vi "ConvertGoop1ToGoop3.vi"() -> (0 "error out":errorcluster)   [LabVIEW 2020]
uses:
  <resource>/Framework/Providers/Open_GDS/ClassProviders/Common/ConvertGoop2ToGoop3_SubVIs/ConvertGoop2ToGoop3_ClassInfo.ctl
  <resource>/Framework/Providers/Open_GDS/ClassProviders/Common/LvClass_class/GDSLvCLass_ClassSettingsType.ctl
  <resource>/Framework/Providers/Open_GDS/ClassProviders/Common/LvClass_class/GDSLvClass_PlugIn.ctl
  <resource>/Framework/Providers/Open_GDS/ClassProviders/Common/LvClass_class/GDSLvClass_PlugInTypes.ctl
  <vilib>/Utility/miscctls.llb/LVPositionTypeDef.ctl
  <vilib>/Utility/error.llb/DialogType.ctl
  <resource>/Framework/Providers/Open_GDS/ClassProviders/Provider_BaseClassInterface/CreateClassData.ctl
  <resource>/Framework/Providers/Open_GDS/ClassProviders/Provider_EndevoGOOP300/Templates/EndevoTemplateNames.ctl
  <resource>/Framework/Providers/Open_GDS/ClassProviders/Provider_EndevoGOOP300/ClassWriterGOOP300_class/ClassWriterGOOP300.lvclass
  <vilib>/picture/picture.llb/imagedata.ctl
  <resource>/Framework/Providers/Open_GDS/ClassProviders/Provider_EndevoGOOP300/EndevoProviderName.ctl
  <vilib>/regexp/Match Regular Expression.xnode
  <resource>/Framework/Providers/Open_GDS/ClassProviders/Provider_BaseClassInterface/ClassWriter_class/ClassWriter.lvclass
panel:
  in  "Cancel":bool
  in  "Next":bool
  out "Tab":T1(tab)
  in  "Current GOOP1 top directory":path
  out "Additional VIs that has been found\nand will be relinked:":i32
  out "GOOP1 classes found":string
  in  "VisToRelink":path[](array[path])
  in  "Project":path caption="This project will be created and have all classes added to it:"
  in  "Progress":i32(listbox)
  in  "Done":bool
  out "State":string
  # "1."
  # "Select Top folder to start a recursive search for GOOP1 classes and application VIs."
  # "2."
  # "These classes\nhave been found.\n\nDo you want to convert them?"
  # "3."
  # "Have you backed up all your VIs in the selected folder?"
  # "Have you checked that all files in\nthe selected folder are writeable?"
  # "Relinking VIs outside top folder?\nIf you want to relink any VIs to the new classes that are outside the selected top folder, add them to the list below"
  # "4."
  # "Save VI dialog boxes!?!\nIt might pop up dialog boxes that asks you to save VIs that will be unloaded from memory, JUST press cancel for those."
  # "Revert dialog boxes!?!\nIt might pop up dialog boxes that prompts that changes has been done on disk, JUST press cancel for those."
  # "5."
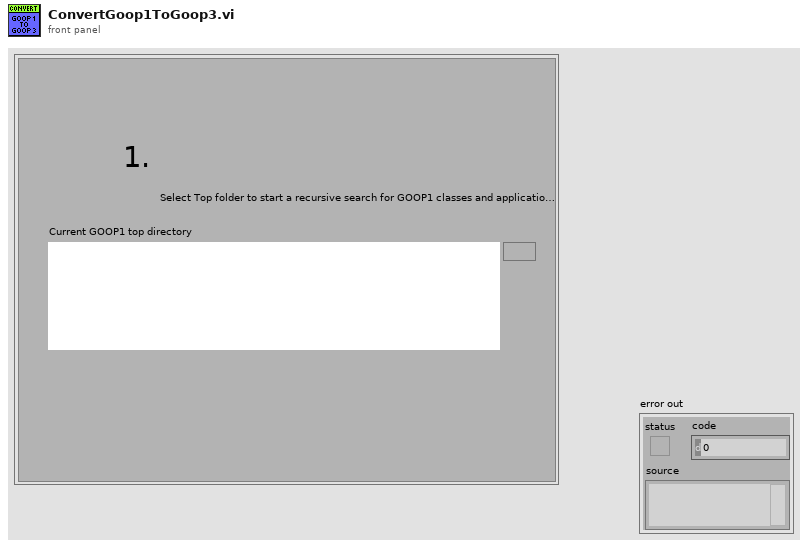
[diagram p1: front panel]
types:
  T1 = enum32{"GOOP2Dir", "ClassesFound", "BackedUp", "Start?", "Converting"}
  T2 = typedef "ConvertGoop2ToGoop3_ClassInfo.ctl" = cluster{"NoOfInheritance":i32, "LvClassPath":path, "ClassName":string, "ClassPrefix":string, "IsLLB":bool, "ClassFolder":path, "ViRefs":refnum<vi>[], "ClassRef":refnum<vi>, "InheritsFrom":path, "RootClass":path, "ViPathes":path[], "AllInheritanceClasses":string[], "TemplateVersionUsed":string, "UsingClassAttributes":bool, "ClassSettings":T3, "HeaderIcon":u8[][]}
  T3 = typedef "GDSLvCLass_ClassSettingsType.ctl" = cluster{"ClassProviderName":string, "ClassTemplateUsed":string, "ClassTemplateVersion":string, "ClassDescription":string, "PlugIns":T4[], "ConnectorPanePattern":string}
  T4 = typedef "GDSLvClass_PlugIn.ctl" = cluster{"Type":T5, "ID":string, "Version":string, "Path":path, "Name":string, "Data":variant}
  T5 = typedef "GDSLvClass_PlugInTypes.ctl" = enum16{"DesignPattern", "MethodTypes"}
  T6 = typedef "LVPositionTypeDef.ctl" = cluster{"Left":i32, "Top":i32}
  T7 = cluster{"TopFolderPath":path, "Classes":T2[], "SetToDynamicDispatch":refnum<vi>[], "error":errorcluster, "Project":path, "ProjectRef":refnum<vi>, "My Computer":refnum<vi>, "AppRef":refnum<vi>, "VIsToRelink":refnum<vi>[], "VIsToRelink(Paths)":path[], "CallParentMethod":cluster{"VIRef":refnum<vi>, "Position":T6}[], "CopyClasses":path, "TemplateVersions":string[], "LLBsToDelete":path[]}
  T8 = enum32{"GOOP2Dir", "ClassesFound", "GOOP3Dir", "Start?", "Converting"}
  T9 = typedef "EndevoTemplateNames.ctl" = enum16{"BaseTemplate", "SubTemplate", "BaseTemplate_4x4x4", "SubTemplate_4x4x4", "SingletonTemplate"}
  T10 = typedef "ClassWriter.lvclass/CreateClassData.ctl" = cluster{"ClassName":string, "ClassFolder":path, "ClassDescription":string, "ClassTemplateOptions":string, "BaseClass(ProjectStringPath or LvClassFilePath)":variant, "ExtraCreateParameters":variant, "FolderSuffix":string}
  T11 = enum32{"invalid scope", "public", "private", "protected"}
  T12 = typedef "imagedata.ctl" = cluster{"image type":i32, "image depth":i32, "image":u8[], "mask":u8[], "colors":u32[], "Rectangle":cluster{"left":i16, "top":i16, "right":i16, "bottom":i16}}
  T13 = typedef "EndevoProviderName.ctl" = enum16{"EndevoGOOP300"}
  T14 = typedef "DialogType.ctl" = u16
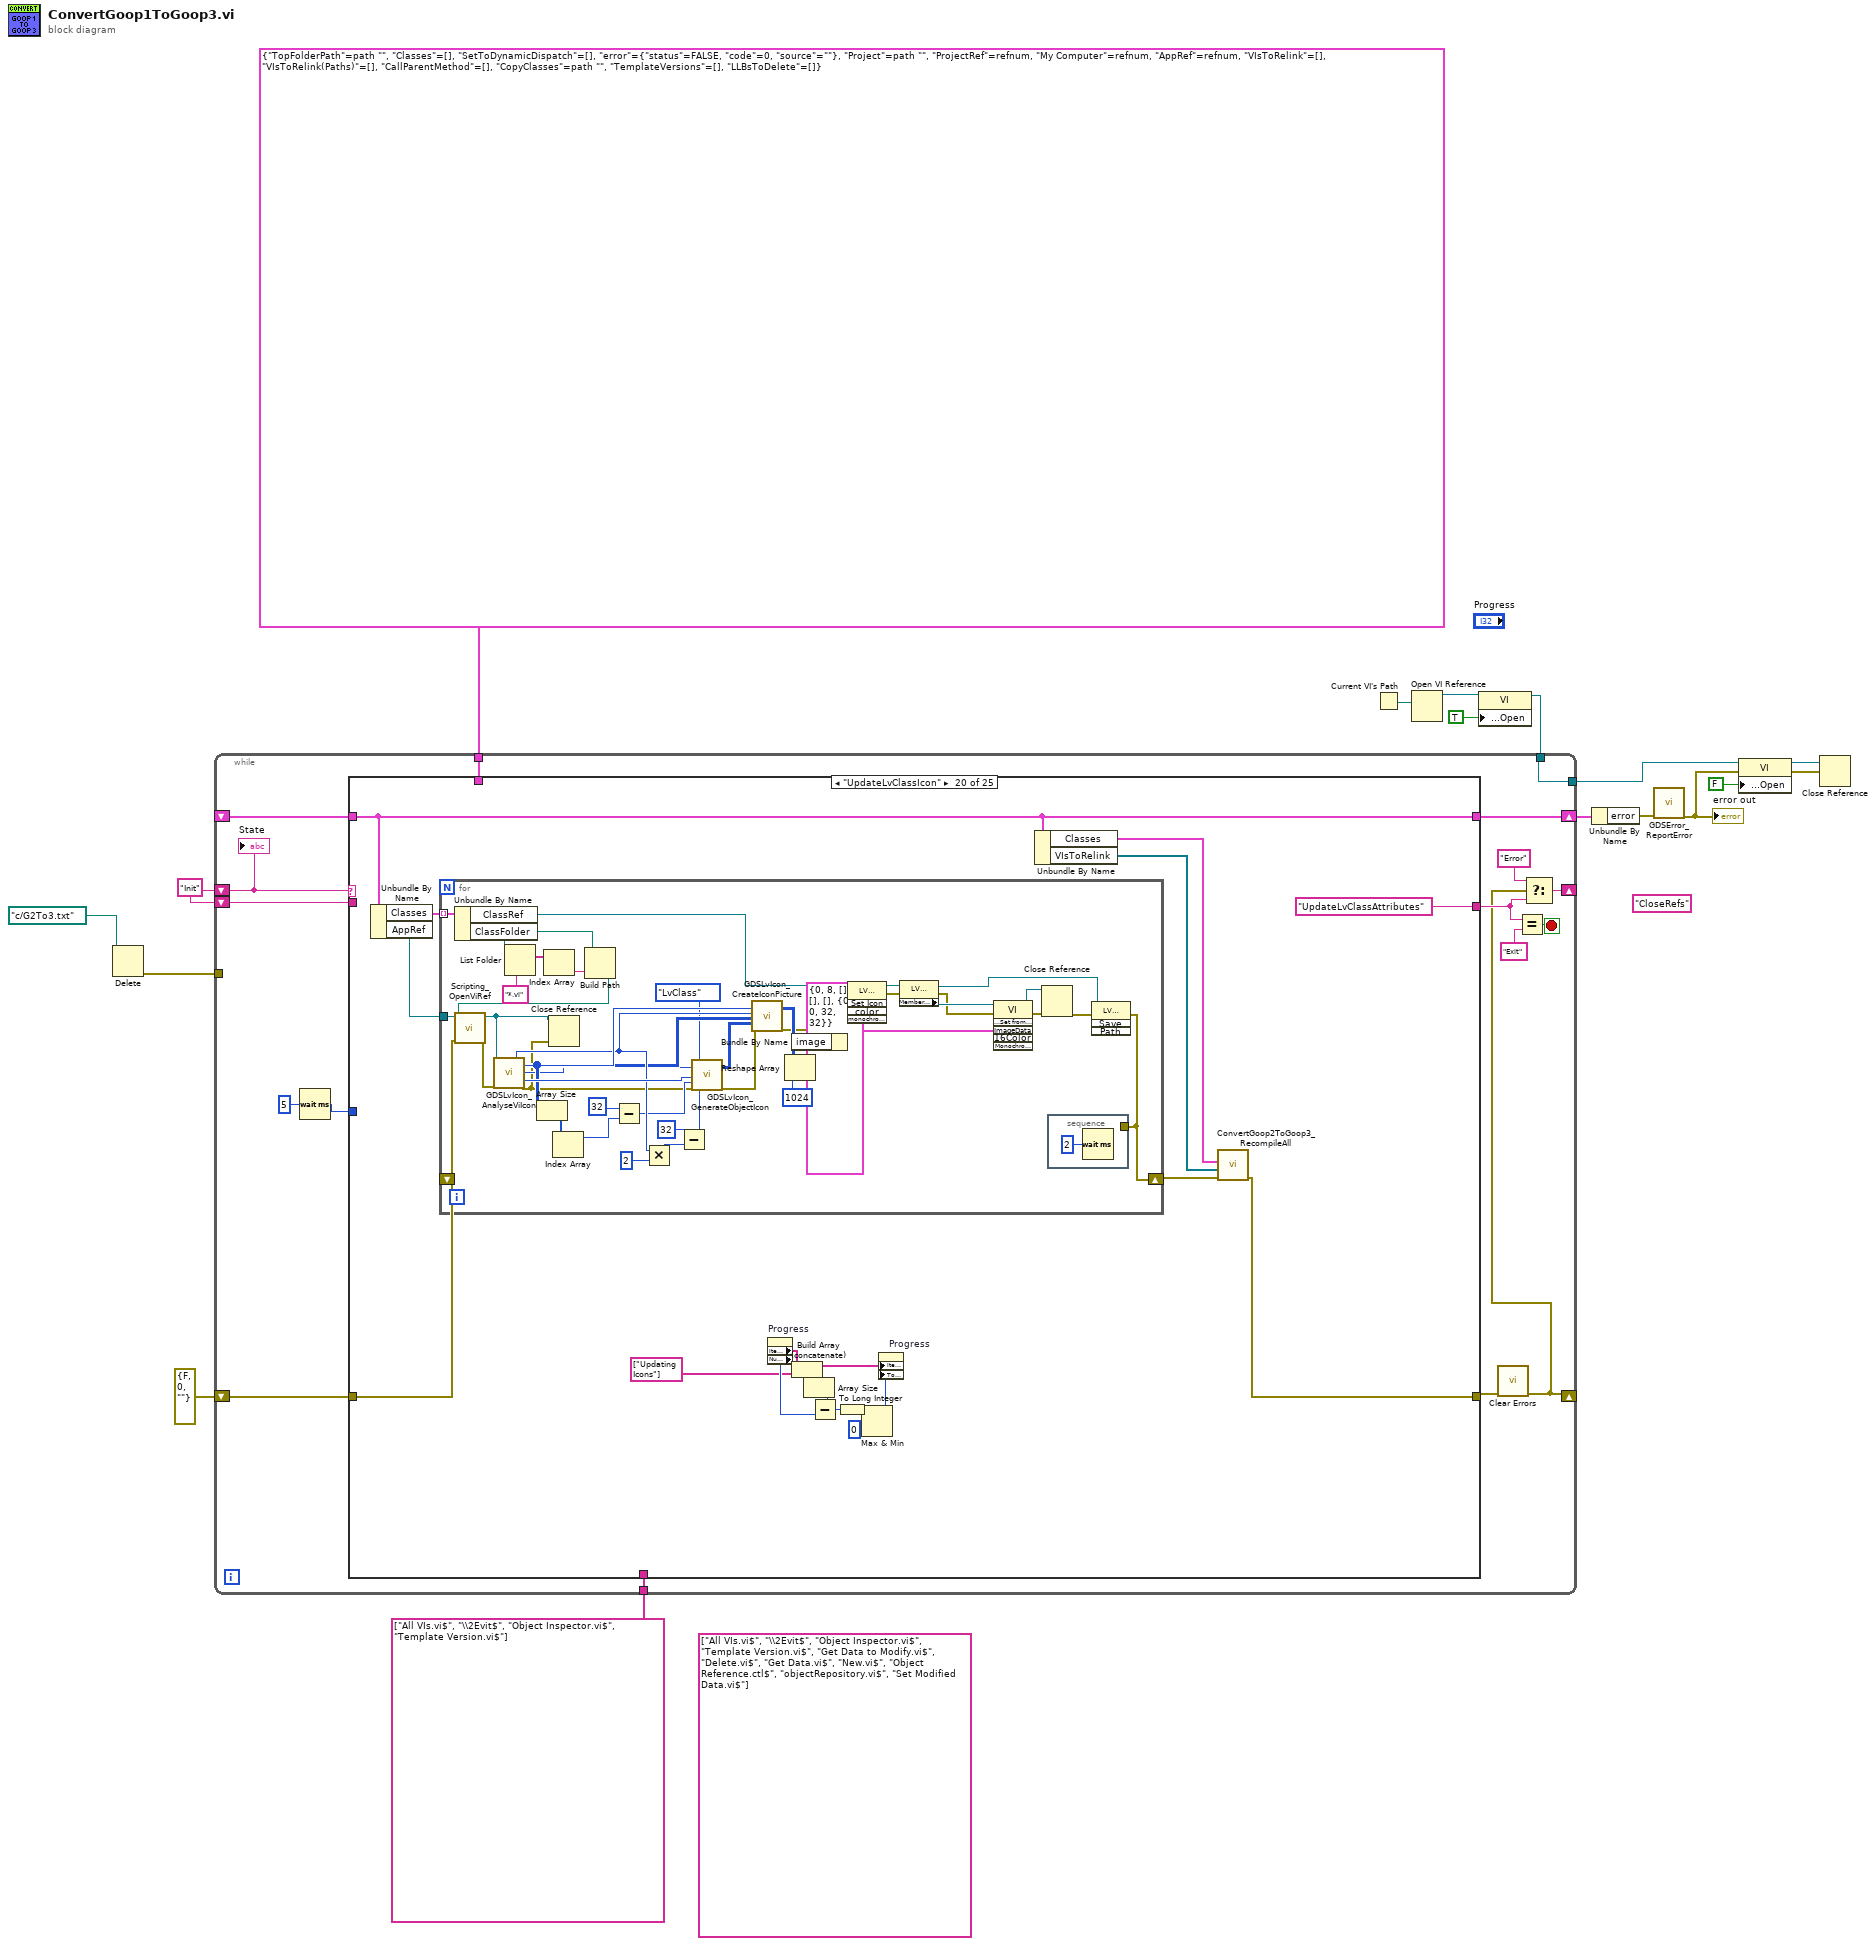
[diagram p0: block diagram]
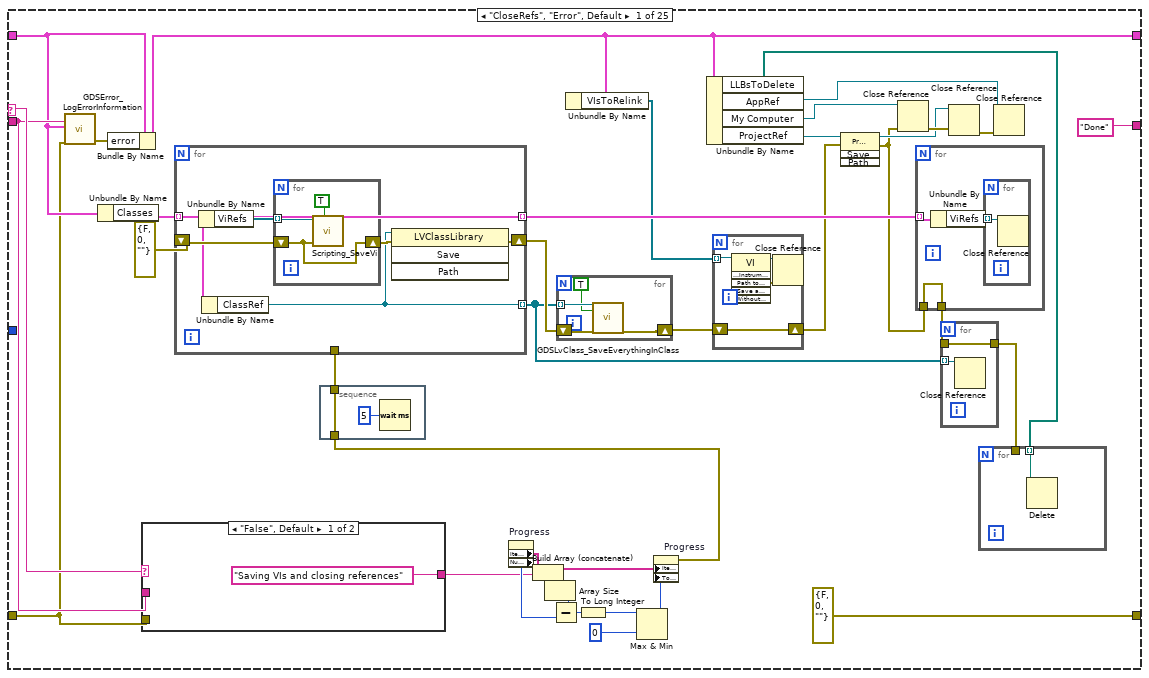
[diagram p2: hidden frame]
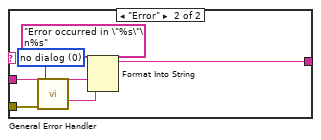
[diagram p3: hidden frame]
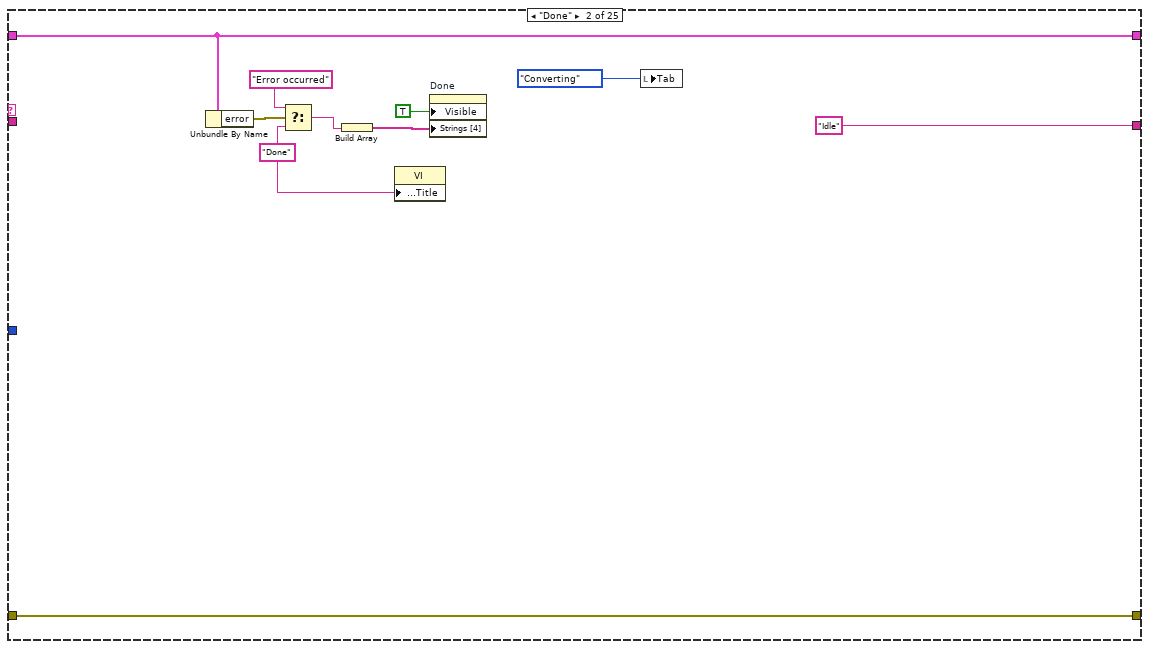
[diagram p4: hidden frame]
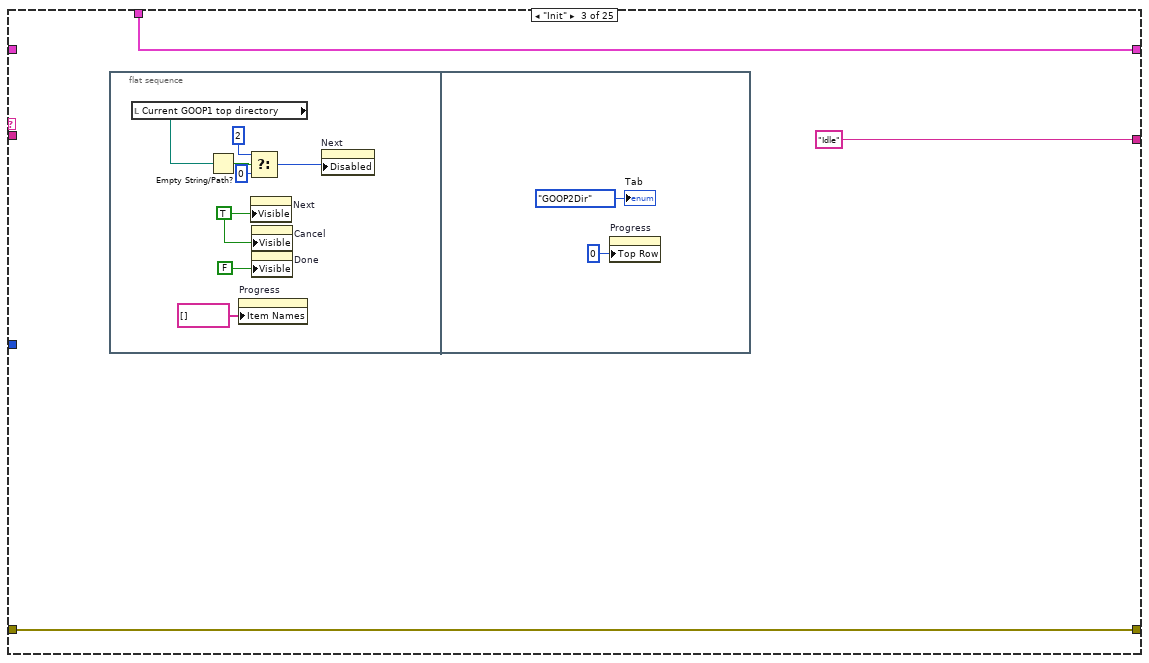
[diagram p5: hidden frame]
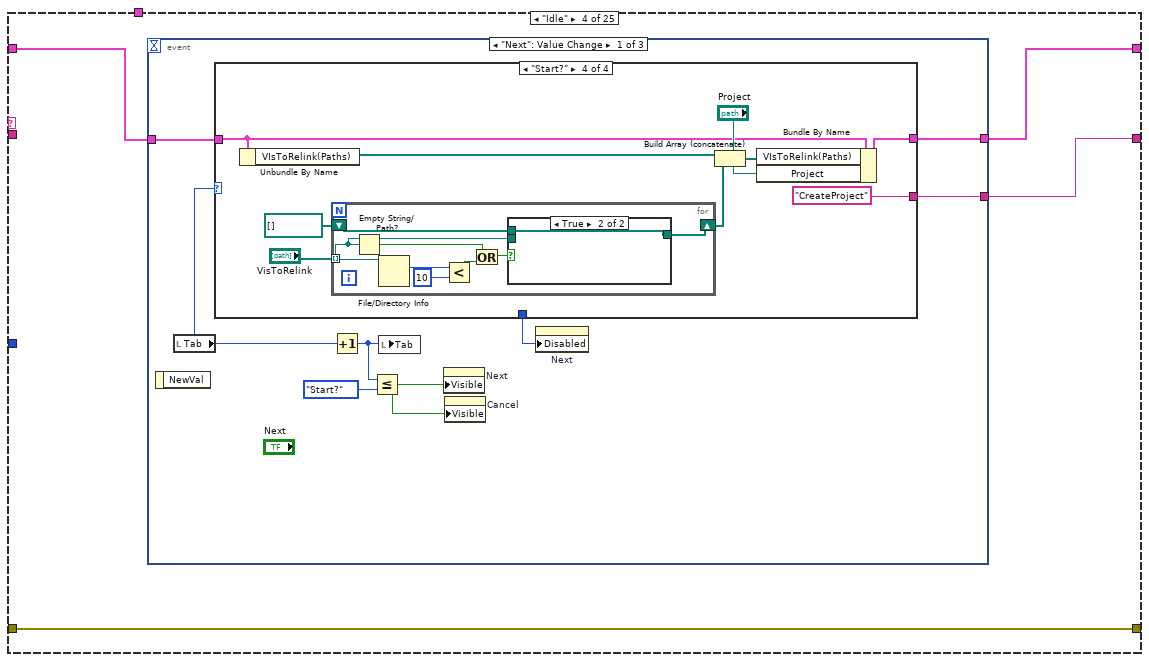
[diagram p6: hidden frame]
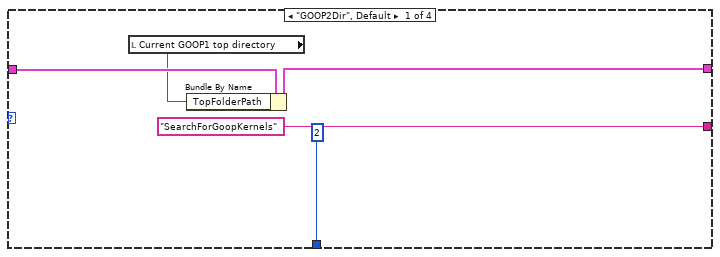
[diagram p7: hidden frame]
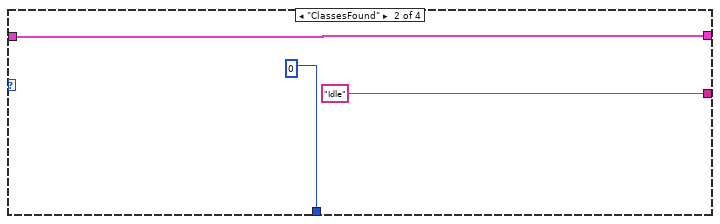
[diagram p8: hidden frame]
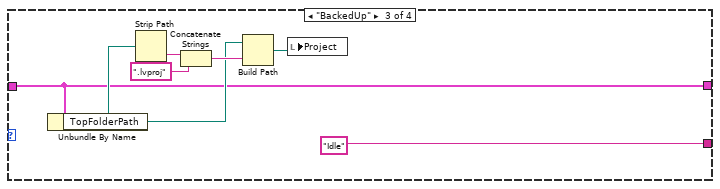
[diagram p9: hidden frame]
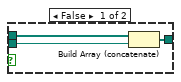
[diagram p10: hidden frame]
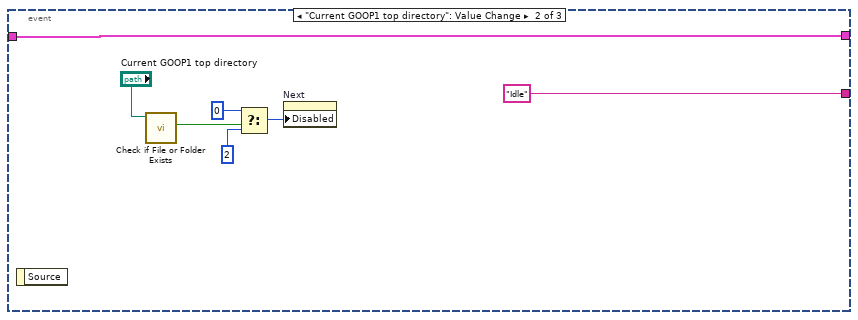
[diagram p11: hidden frame]
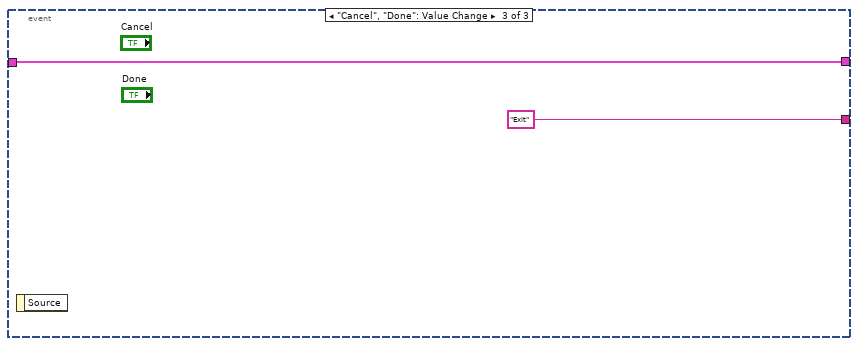
[diagram p12: hidden frame]
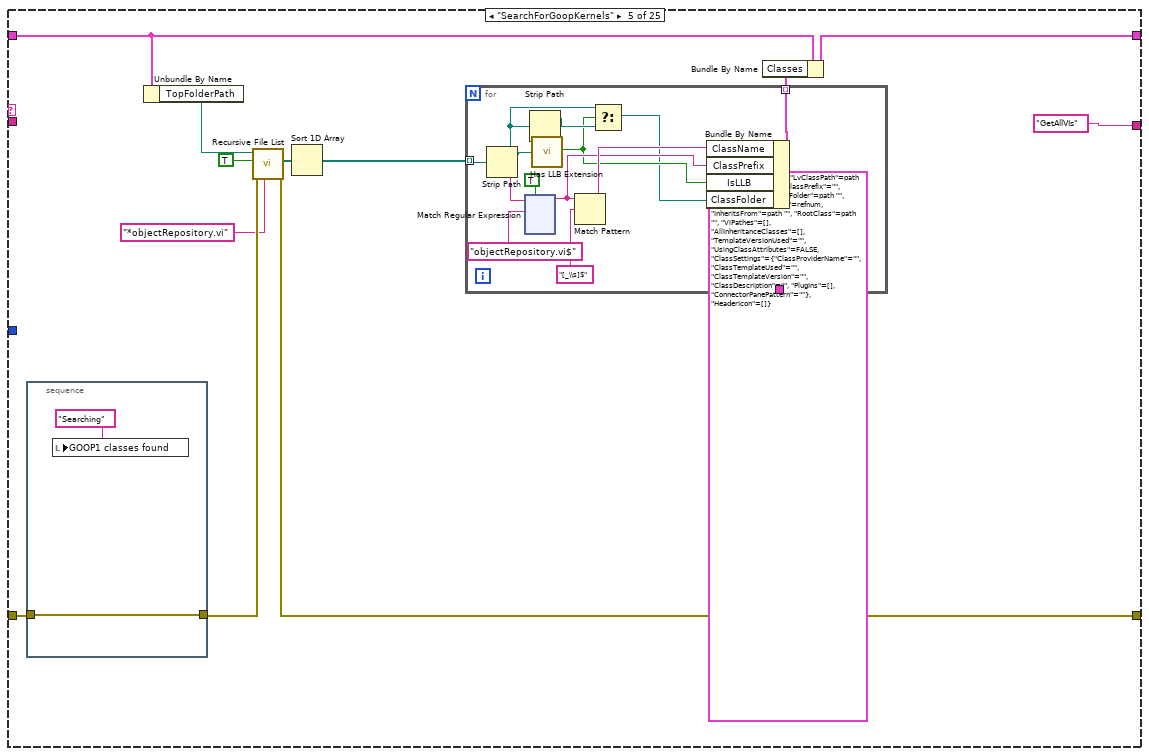
[diagram p13: hidden frame]
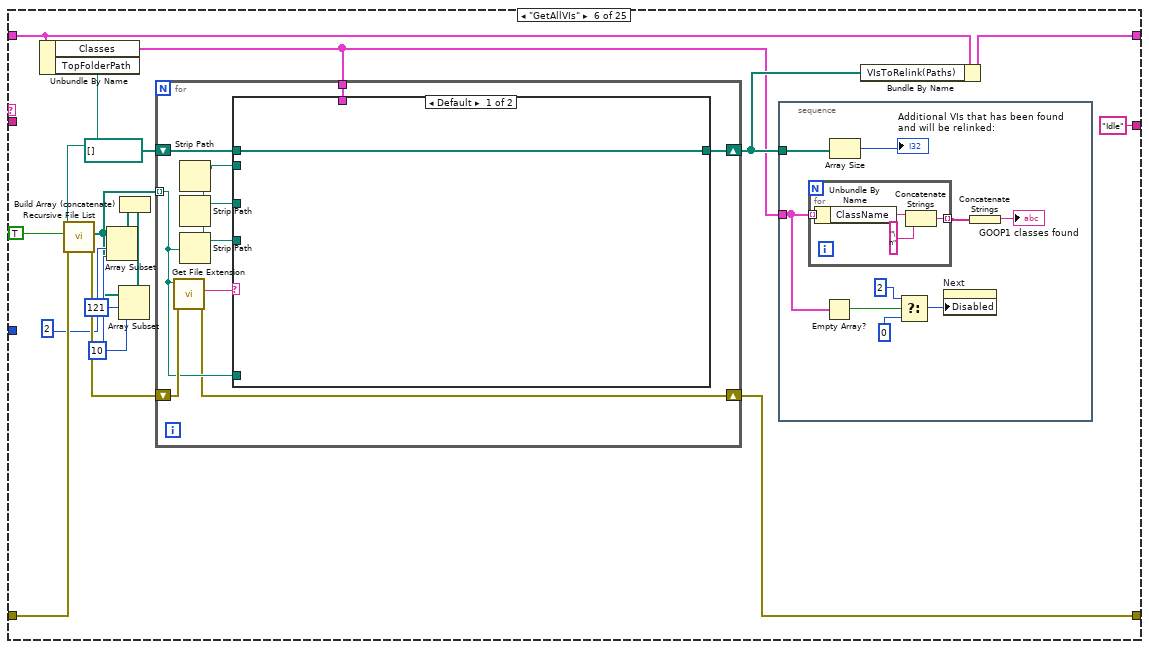
[diagram p14: hidden frame]
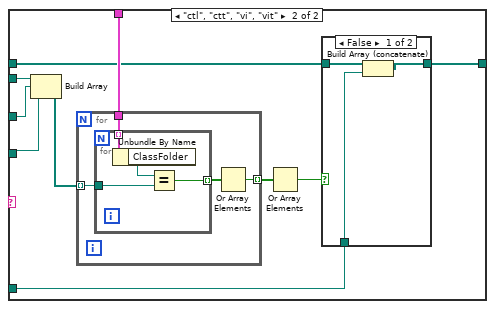
[diagram p15: hidden frame]
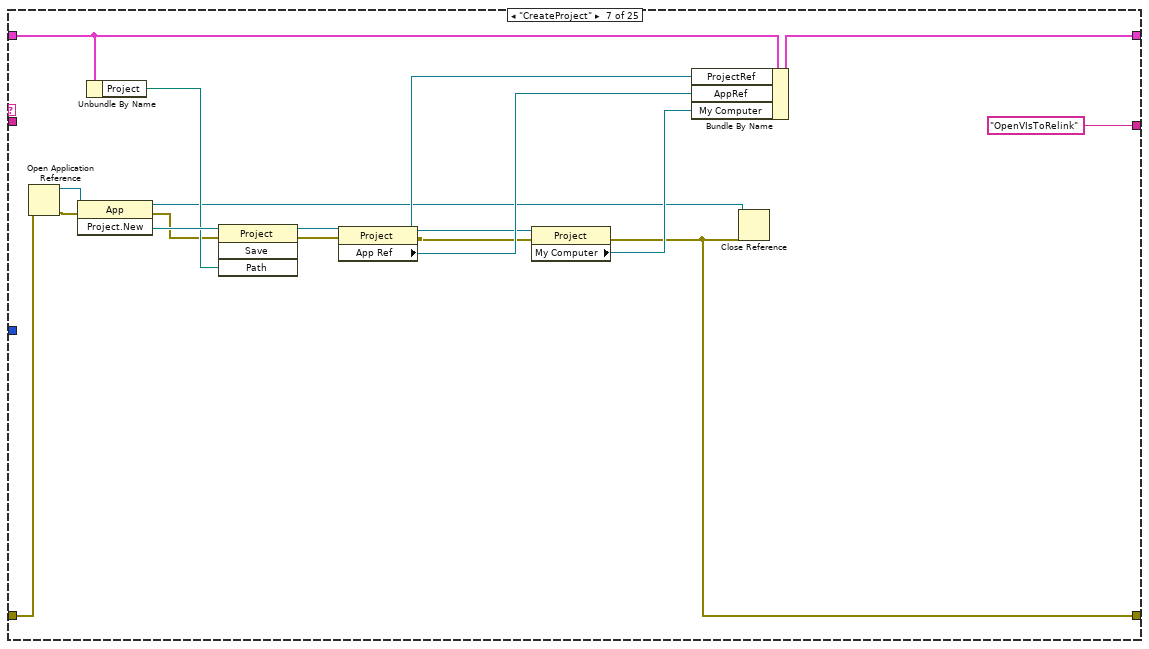
[diagram p17: hidden frame]
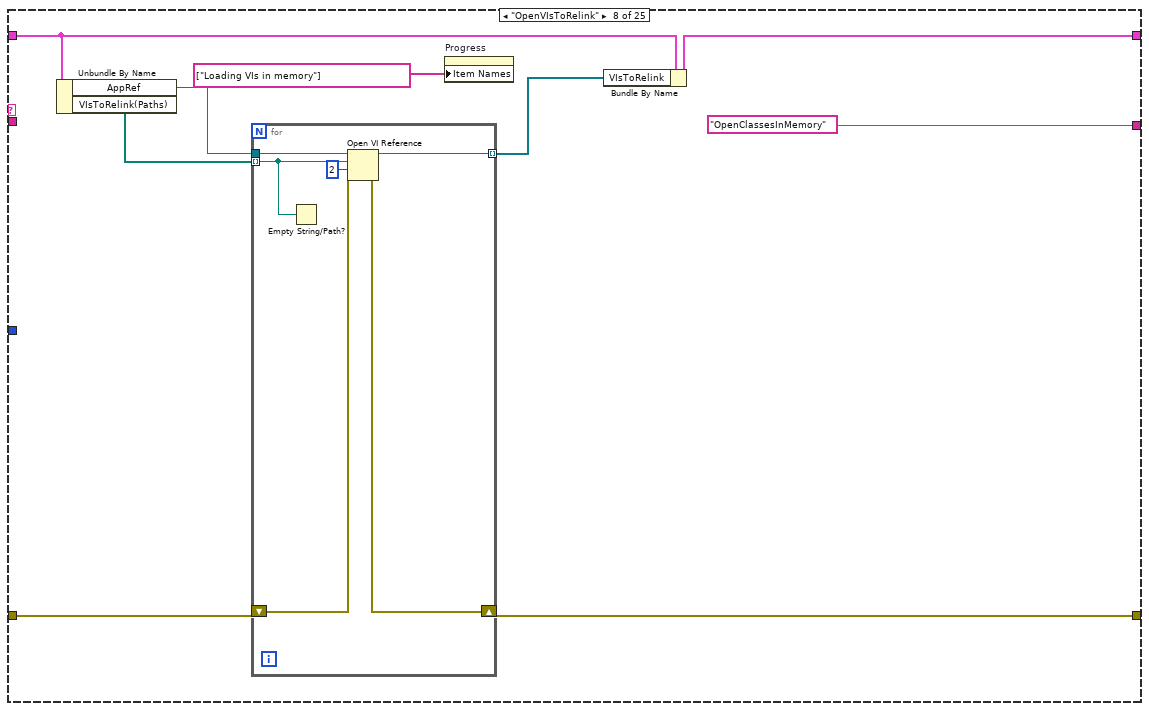
[diagram p18: hidden frame]
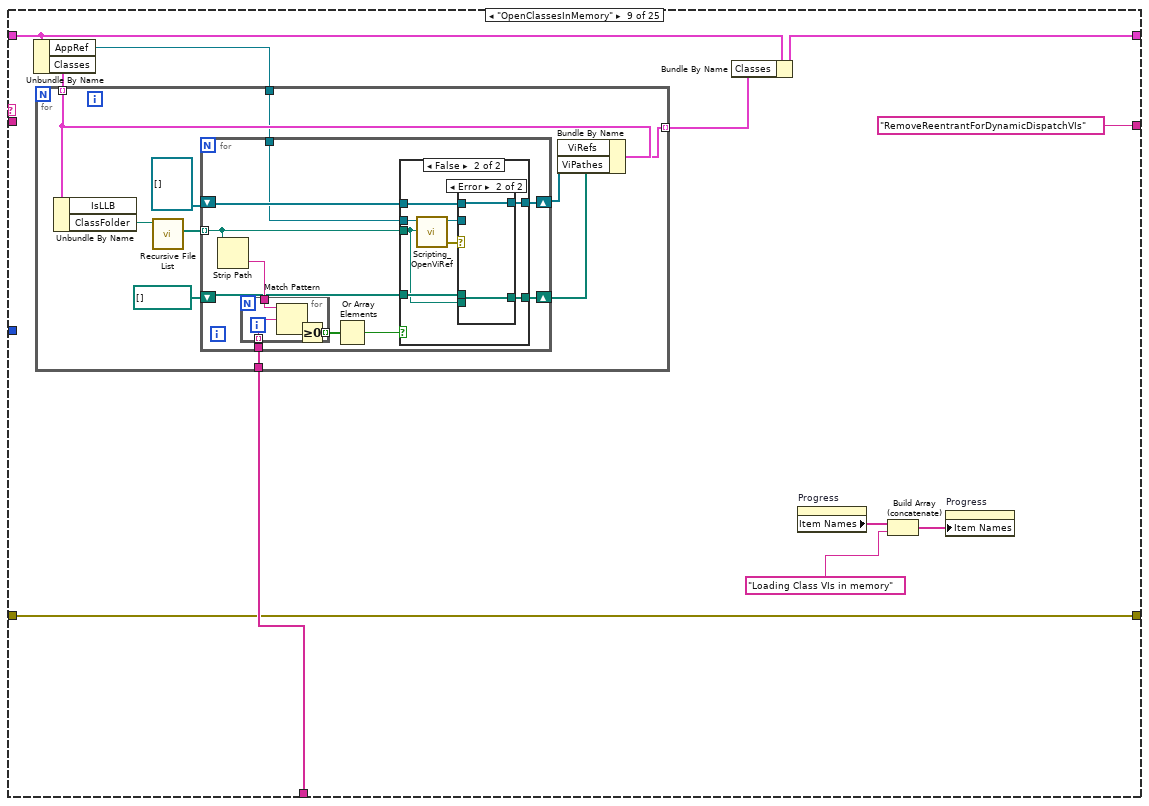
[diagram p19: hidden frame]
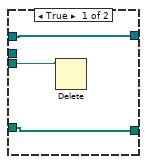
[diagram p20: hidden frame]
diagram:
  (unwired) "CloseRefs"
  (unwired) string[] ["All VIs.vi$", "\\2Evit$", "Object Inspector.vi$", "Template Version.vi$", "Get Data to Modify.vi$", "Delete.vi$", "Get Data.vi$", "New.vi$", "Object Reference.ctl$", "objectRepository.vi$", "Set Modified Data.vi$"] ("file names")
  w14 = "Init"
  n1 = Delete(path (use dialog)=path "c:/G2To3.txt" ("file (use dialog)")) -> (error out=w11:errorcluster)  [unwired: 4 in, 2 out]
  n2 = Current VI's Path() -> (path=w9:path)
  n3 = Open VI Reference(vi path=w9) -> (vi reference=w8:refnum<vi>)  [unwired: 5 in, 1 out]
  n4 = property class="VI"(reference=w8, "Front Panel.Open"=TRUE ("Front Panel Window:Open")) -> (reference out=w7:refnum<vi>)  [unwired: 1 in, 1 out]
  n5 = while {
    shift-right: [w18] -> _
    shift-left: errorcluster {"status"=FALSE, "code"=0, "source"=""} ("error IO") -> [w34]
    shift-right: [w33] -> _
    shift-left: w14 -> [w23]
    shift-right: [w28] -> w13
    shift-left: _ -> [w27]
    tunnel: T7 {"TopFolderPath"=path "", "Classes"=[], "SetToDynamicDispatch"=[], "error"={"status"=FALSE, "code"=0, "source"=""}, "Project"=path "", "ProjectRef"=refnum, "My Computer"=refnum, "AppRef"=refnum, "VIsToRelink"=[], "VIsToRelink(Paths)"=[], "CallParentMethod"=[], "CopyClasses"=path "", "TemplateVersions"=[], "LLBsToDelete"=[]} -> [w26]
    tunnel: string[] ["All VIs.vi$", "\\2Evit$", "Object Inspector.vi$", "Template Version.vi$"] ("file names") -> [w25]
    shift-left: w14 -> [w24]
    tunnel: w11 -> [_]
    tunnel: w7 -> [w20]
    tunnel: [w20] -> w2
    stop <- w32 stop-if-true
    n6 = Wait (ms)(milliseconds to wait=u32 5) -> (millisecond timer value=w21:u32)
    n7 = case shown="\"UpdateLvClassIcon\"" w23 {
      selector: w23 -> [w66 _ _ _ _ _ _ _ _ _ _ _ _ _ _ _ _ _ _ _ _ _ _ _ _]
      tunnel: w34 -> [w60 w113 w116 w128 w191 w337 w397 w409 w425 w476 w521 w531 w572 w712 w773 w818 w872 w946 w989 w1126 w1177 w1219 w1256 w1282 w1366]
      tunnel: [errorcluster {"status"=FALSE, "code"=0, "source"=""} ("error IO") w113 w116 w128 w195 w335 w388 w408 w425 w475 w520 w527 w573 w713 w747 w810 w868 w943 w988 w1113 w1175 w1221 w1258 w1281 w1365] -> w19
      tunnel: ["Done" "Idle" "Idle" w129 "GetAllVIs" "Idle" "OpenVIsToRelink" "OpenClassesInMemory" "RemoveReentrantForDynamicDispatchVIs" "RecompilingVIs" "AddVIsToProject" "RenameFiles" "RenameTempNames" "CreateCopyClasses" "UpdateVIsGoopRefs" "CopyVIsOver" "RelinkAllSubVIs" "ConnectVIsToClass" "UpdateLvClassIcon" "UpdateLvClassAttributes" "UpdateNewCallers" "UpdateDeleteCallers" "UpdateConnectorPane" "UpdateClassInfo" "CloseRefs"] -> w29
      tunnel: [w49 w112 w115 w130 w193 w333 w399 w411 w427 w477 w513 w524 w571 w711 w753 w812 w869 w944 w987 w1111 w1174 w1220 w1257 w1279 w1364] -> w28
      tunnel: w27 -> [w62 w112 _ w131 w194 w334 w401 w412 w428 w477 w513 w524 w566 w711 w754 w812 w869 w944 w987 w1111 w1174 w1220 w1257 w1279 w1364]
      tunnel: w26 -> [_ _ w115 _ _ _ _ _ _ _ _ _ _ _ _ _ _ _ _ _ _ _ _ _ _]
      tunnel: w25 -> [_ _ _ _ _ _ _ _ w426 _ _ _ _ _ _ _ _ _ _ _ _ _ _ _ _]
      tunnel: w24 -> [w65 _ _ _ _ _ _ _ _ _ _ _ _ _ _ _ _ _ _ _ _ _ _ _ _]
      tunnel: w21 -> [_ _ _ _ _ _ _ _ _ _ _ _ _ _ _ _ _ _ _ _ _ _ _ _ _]
      frame "CloseRefs", "Error", Default {
        n8 = call <resource>:"GDSError_LogErrorInformation.vi"("State"=w65, "LocalVariableData"=w62, "error in (no error)"=w60) -> ("error out"=w52:errorcluster)  [unwired: 16 in]
        n9 = Unbundle By Name(w62) -> ("Classes"=w70:T2[])
        n10 = Bundle By Name(cluster=w62, "error"=w52) -> (w49:T7)
        n11 = case shown="\"False\", Default" w66 {
          tunnel: w65 -> [_ w84]
          tunnel: w60 -> [_ w82]
          tunnel: ["Saving VIs and closing references" w80] -> w39
          frame "False", Default {
          }
          frame "Error" {
            w83 = T14 0 items=["no dialog", "OK message", "continue or stop message", "OK message + warnings", "continue/stop + warnings"] ("type of dialog (OK msg:1)")
            n12 = call <vilib>:"General Error Handler.vi"("type of dialog (OK msg:1)"=w83, "error in (no error)"=w82) -> ("message"=w81:string)  [unwired: 9 in, 4 out]
            n13 = Format Into String(format string="Error occurred in \"%s\"\n%s", w84, w81) -> (resulting string=w80:string)  [unwired: 2 in, 1 out]
          }
        }
        n14 = property on="Progress" class="LstBox (strict)"() -> ("Item Names"=w47:string[], "Number of Rows"=w41:u32)  [unwired: 2 in, 2 out]
        n15 = Build Array (concatenate)(w47, w39) -> (w42:string[])
        n16 = Array Size(array=w42) -> (size(s)=w46:i32)
        n17 = Subtract(x=w46, y=w41) -> (x-y=w45:u32)
        n18 = Unbundle By Name(w49) -> ("VIsToRelink"=w54:refnum<vi>[])
        n19 = To Long Integer(number=w45) -> (32bit integer=w43:i32)
        n20 = Max & Min(x=w43, y=0) -> (max(x,y)=w40:i32)  [unwired: 1 out]
        n21 = property on="Progress" class="LstBox (strict)"("Item Names"=w42, "Top Row"=w40) -> (error out=w38:errorcluster)  [unwired: 2 in, 1 out]
        n22 = stacked-sequence {
          tunnel: w38 -> [w73]
          tunnel: [w73] -> w37
          frame #0 {
            n23 = Wait (ms)(milliseconds to wait=u32 5) -> ()  [unwired: 1 out]
          }
        }
        n24 = for {
          tunnel: w70 -> [w99] mode=indexing
          tunnel: [w99] -> w69 mode=indexing
          shift-right: [w97] -> w68
          shift-left: errorcluster {"status"=FALSE, "code"=0, "source"=""} ("error out") -> [w100]
          tunnel: [w96] -> w67 mode=indexing
          tunnel: w37 -> [_]
          n25 = Unbundle By Name(w99) -> ("ViRefs"=w101:refnum<vi>[])
          n26 = Unbundle By Name(w99) -> ("ClassRef"=w96:refnum<vi>)
          n27 = for {
            tunnel: w101 -> [w104] mode=indexing
            shift-right: [w102] -> w98
            shift-left: w100 -> [w102]
            n28 = call <resource>:"Scripting_SaveVi.vi"("ForceResaving(False)"=TRUE, "error in (no error)"=w102, "VIRefToSaveIn"=w104) -> ()  [unwired: 7 in, 2 out]
          }
          n29 = invoke class="LVClassLibrary" method="Save"(reference=w96, error in=w98) -> (error out=w97:errorcluster)  [unwired: 2 in, 3 out]
        }
        n30 = for {
          shift-right: [w90] -> w51
          shift-left: w68 -> [w91]
          tunnel: w67 -> [w89] mode=indexing
          n31 = call <resource>:"GDSLvClass_SaveEverythingInClass.vi"("ClassRefIn"=w89, "ForceResaving(False)"=TRUE, "error in"=w91) -> ("error out"=w90:errorcluster)  [unwired: 15 in, 1 out]
        }
        n32 = Unbundle By Name(w49) -> ("LLBsToDelete"=w35:path[], "AppRef"=w55:refnum<vi>, "My Computer"=w48:refnum<vi>, "ProjectRef"=w59:refnum<vi>)
        n33 = for {
          tunnel: w54 -> [w76] mode=indexing
          shift-right: [w75] -> w50
          shift-left: w51 -> [w75]
          n34 = invoke class="VI" method="Save.Instrument"(reference=w76) -> (reference out=w77:refnum<vi>, error out=w78:errorcluster)  [unwired: 5 in, 4 out]
          n35 = Close Reference(reference=w77, error in (no error)=w78) -> ()  [unwired: 1 out]
        }
        n36 = invoke class="Project" method="Save"(reference=w59, error in=w50) -> (reference out=w57:refnum<vi>, error out=w53:errorcluster)  [unwired: 2 in, 2 out]
        n37 = Close Reference(reference=w48, error in (no error)=w53) -> (error out=w58:errorcluster)
        n38 = for {
          tunnel: w69 -> [w94] mode=indexing
          tunnel: w53 -> [w92]
          tunnel: [w92] -> w64
          n39 = Unbundle By Name(w94) -> ("ViRefs"=w93:refnum<vi>[])
          n40 = for {
            tunnel: w93 -> [w95] mode=indexing
            n41 = Close Reference(reference=w95) -> ()  [unwired: 1 in, 1 out]
          }
        }
        n42 = for {
          tunnel: w67 -> [w87] mode=indexing
          tunnel: w64 -> [w86]
          tunnel: [w86] -> w36
          n43 = Close Reference(reference=w87) -> ()  [unwired: 1 in, 1 out]
        }
        n44 = Close Reference(reference=w57, error in (no error)=w58) -> (error out=w56:errorcluster)
        n45 = for {
          tunnel: w36 -> [_]
          tunnel: w35 -> [w72] mode=indexing
          n46 = Delete(path (use dialog)=w72) -> ()  [unwired: 4 in, 3 out]
        }
        n47 = Close Reference(reference=w55, error in (no error)=w56) -> ()  [unwired: 1 out]
      }
      frame "Done" {
        w105 = "Done"
        n48 = Unbundle By Name(w112) -> ("error"=w111:errorcluster)
        n49 = Select(t="Error occurred", s=w111, f=w105) -> (s? t:f=w108:string)
        n50 = Build Array(w108) -> (w107:string[])
        n51 = property class="VI"("Front Panel.Title"=w105) -> ()  [unwired: 2 in, 2 out]
        n52 = property on="Done" class="Bool"("Visible"=TRUE, "Strings [4]"=w107) -> ()  [unwired: 2 in, 2 out]
        n53 = local write "Tab"(T1."Converting" ("Tab")) -> ()
      }
      frame "Init" {
        n54 = flat-sequence {
          frame #0 {
            w125 = TRUE ("Visible")
            n55 = local read "Current GOOP1 top directory"() -> (w122:path)
            n56 = Empty String/Path?(string/path=w122) -> (empty?=w121:bool)
            n57 = property on="Progress" class="LstBox (strict)"("Item Names"=string[] []) -> ()  [unwired: 2 in, 2 out]
            n58 = Select(t=u8 2 ("Disabled"), s=w121, f=u8 0) -> (s? t:f=w119:u8)
            n59 = property on="Next" class="Bool"("Visible"=w125) -> ()  [unwired: 2 in, 2 out]
            n60 = property on="Cancel" class="Bool"("Visible"=w125) -> ()  [unwired: 2 in, 2 out]
            n61 = property on="Done" class="Bool"("Visible"=FALSE) -> ()  [unwired: 2 in, 2 out]
            n62 = property on="Next" class="Bool"("Disabled"=w119) -> ()  [unwired: 2 in, 2 out]
          }
          frame #1 {
            n63 = property on="Progress" class="LstBox (strict)"("Top Row"=0) -> ()  [unwired: 2 in, 2 out]
            "Tab" <- T1."GOOP2Dir" ("Tab")
          }
        }
      }
      frame "Idle" {
        n64 = event shown="[0] \"Next\": Value Change" {
          selector: _ -> [_ _ _]
          dyn-events: _ -> [_ _ _]
          timeout: _ -> [_ _ _]
          tunnel: w131 -> [w135 w178 w183]
          tunnel: [w134 w178 w183] -> w130
          tunnel: [w133 "Idle" "Exit"] -> w129
          event "Next": Value Change {
            n65 = event-data() -> ()  [unwired: 1 in, 1 out]
            n66 = local read "Tab"() -> (w136:T1)
            n67 = case shown="\"Start?\"" w136 {
              tunnel: w135 -> [w144 w146 w149 w160]
              tunnel: [w143 w146 w149 w163] -> w134
              tunnel: ["SearchForGoopKernels" "Idle" "Idle" "CreateProject"] -> w133
              tunnel: [u8 2 ("Disabled") u8 0 ("f") _ _] -> w132
              frame "GOOP2Dir", Default {
                n68 = local read "Current GOOP1 top directory"() -> (w141:path)
                n69 = Bundle By Name(cluster=w144, "TopFolderPath"=w141) -> (w143:T7)
              }
              frame "ClassesFound" {
              }
              frame "BackedUp" {
                n70 = Unbundle By Name(w149) -> ("TopFolderPath"=w150:path)
                n71 = Strip Path(path=w150) -> (name=w153:string)  [unwired: 1 out]
                n72 = Concatenate Strings(w153, ".lvproj" ("string")) -> (w151:string)
                n73 = Build Path(base path=w150, name or relative path=w151) -> (appended path=w148:path)
                n74 = local write "Project"(w148) -> ()
              }
              frame "Start?" {
                n75 = Unbundle By Name(w160) -> ("VIsToRelink(Paths)"=w159:path[])
                n76 = for {
                  tunnel: "VisToRelink" -> [w165] mode=indexing
                  shift-right: [w164] -> w155
                  shift-left: path[] [] -> [w166]
                  n77 = Empty String/Path?(string/path=w165) -> (empty?=w168:bool)
                  n78 = File/Directory Info(path=w165) -> (size=w171:i64)  [unwired: 1 in, 6 out]
                  n79 = Less?(x=w171, y=i64 10) -> (x < y?=w169:bool)
                  n80 = Or(x=w168, y=w169) -> (x .or. y?=w167:bool)
                  n81 = case shown="True" w167 {
                    tunnel: w166 -> [w174 w175]
                    tunnel: w165 -> [w173 _]
                    tunnel: [w172 w175] -> w164
                    frame False {
                      n82 = Build Array (concatenate)(w174, w173) -> (w172:path[])
                    }
                    frame True {
                    }
                  }
                }
                n83 = Build Array (concatenate)(w159, w155) -> (w158:path[])
                n84 = Bundle By Name(cluster=w160, "VIsToRelink(Paths)"=w158, "Project"="Project") -> (w163:T7)
              }
            }
            n85 = Increment(x=w136) -> (x+1=w139:T1)
            n86 = Less Or Equal?(x=w139, y=T8."Start?") -> (x <= y?=w137:bool)
            n87 = local write "Tab"(w139) -> ()
            n88 = property on="Next" class="Bool"("Visible"=w137) -> ()  [unwired: 2 in, 2 out]
            n89 = property on="Cancel" class="Bool"("Visible"=w137) -> ()  [unwired: 2 in, 2 out]
            n90 = property on="Next" class="Bool"("Disabled"=w132) -> ()  [unwired: 2 in, 2 out]
          }
          event "Current GOOP1 top directory": Value Change {
            n91 = event-data() -> ()  [unwired: 1 in, 1 out]
            n92 = call <vilib>:"Check if File or Folder Exists.vi"("path"="Current GOOP1 top directory") -> ("file or folder exists?"=w182:bool)  [unwired: 8 in, 2 out]
            n93 = Select(t=u8 0, s=w182, f=u8 2 ("Disabled")) -> (s? t:f=w181:u8)
            n94 = property on="Next" class="Bool"("Disabled"=w181) -> ()  [unwired: 2 in, 2 out]
          }
          event "Cancel", "Done": Value Change {
            n95 = event-data() -> ()  [unwired: 1 in, 1 out]
          }
        }
      }
      frame "SearchForGoopKernels" {
        n96 = stacked-sequence {
          tunnel: w191 -> [w198]
          tunnel: [w198] -> w190
          frame #0 {
            n97 = local write "GOOP1 classes found"("Searching" ("GOOP2 classes found")) -> ()
          }
        }
        n98 = Unbundle By Name(w194) -> ("TopFolderPath"=w197:path)
        n99 = call <vilib>:"Recursive File List.vi"("pattern"="*objectRepository.vi", "error in (no error)"=w190, "Treat LLBs as Folders?"=TRUE, "Folder Path"=w197) -> ("error out"=w195:errorcluster, "All Files in Dir"=w189:path[])  [unwired: 3 in, 3 out]
        n100 = Sort 1D Array(array=w189) -> (sorted array=w187:path[])
        n101 = for {
          tunnel: w187 -> [w212] mode=indexing
          tunnel: T2 {"NoOfInheritance"=0, "LvClassPath"=path "", "ClassName"="", "ClassPrefix"="", "IsLLB"=FALSE, "ClassFolder"=path "", "ViRefs"=[], "ClassRef"=refnum, "InheritsFrom"=path "", "RootClass"=path "", "ViPathes"=[], "AllInheritanceClasses"=[], "TemplateVersionUsed"="", "UsingClassAttributes"=FALSE, "ClassSettings"={"ClassProviderName"="", "ClassTemplateUsed"="", "ClassTemplateVersion"="", "ClassDescription"="", "PlugIns"=[], "ConnectorPanePattern"=""}, "HeaderIcon"=[]} ("output cluster") -> [w206]
          tunnel: [w201] -> w186 mode=indexing
          n102 = Strip Path(path=w212) -> (stripped path=w208:path, name=w211:string)
          n103 = xnode "Match Regular Expression"("input string"=w211, "regular expression"="objectRepository.vi$", "ignore case? (F)"=TRUE) -> ("before match"=w204:string)  [unwired: 3 in, 4 out]
          n104 = Strip Path(path=w208) -> (stripped path=w207:path)  [unwired: 1 out]
          n105 = call <vilib>:"Has LLB Extension.vi"("path"=w208) -> ("path to VI library?"=w203:bool)
          n106 = Match Pattern(string=w204, regular expression="[_\\s]$") -> (before substring=w205:string)  [unwired: 1 in, 3 out]
          n107 = Select(t=w208, s=w203, f=w207) -> (s? t:f=w202:path)
          n108 = Bundle By Name(cluster=w206, "ClassName"=w205, "ClassPrefix"=w204, "IsLLB"=w203, "ClassFolder"=w202) -> (w201:T2)
        }
        n109 = Bundle By Name(cluster=w194, "Classes"=w186) -> (w193:T7)
      }
      frame "GetAllVIs" {
        w328 = 10 ("length")
        n110 = Unbundle By Name(w334) -> ("Classes"=w331:T2[], "TopFolderPath"=w340:path)
        n111 = call <vilib>:"Recursive File List.vi"("error in (no error)"=w337, "Treat LLBs as Folders?"=TRUE, "Folder Path"=w340) -> ("error out"=w336:errorcluster, "All Files in Dir"=w324:path[])  [unwired: 4 in, 3 out]
        n112 = Array Subset(array=w324, index=2, length=w328) -> (w326:path[])
        n113 = Array Subset(array=w324, index=121, length=w328) -> (w325:path[])
        n114 = Build Array (concatenate)(w326, w325) -> ()  [unwired: 1 out]
        n115 = for {
          shift-right: [w362] -> w332
          shift-left: path[] [] ("All Files in Dir") -> [w361]
          tunnel: w324 -> [w355] mode=indexing
          shift-right: [w354] -> w335
          shift-left: w336 -> [w360]
          tunnel: w331 -> [w356]
          n116 = call <vilib>:"Get File Extension.vi"("error in (no error)"=w360, "file"=w355) -> ("error out"=w354:errorcluster, "lowercase file extension"=w363:string)  [unwired: 5 in, 3 out]
          n117 = Strip Path(path=w355) -> (stripped path=w359:path)  [unwired: 1 out]
          n118 = Strip Path(path=w359) -> (stripped path=w357:path)  [unwired: 1 out]
          n119 = Strip Path(path=w357) -> (stripped path=w358:path)  [unwired: 1 out]
          n120 = case shown="Default" w363 {
            tunnel: [w364 w367] -> w362
            tunnel: w361 -> [w364 w366]
            tunnel: w359 -> [_ w372]
            tunnel: w358 -> [_ w374]
            tunnel: w357 -> [_ w373]
            tunnel: w356 -> [_ w370]
            tunnel: w355 -> [_ w365]
            frame Default {
            }
            frame "ctl", "ctt", "vi", "vit" {
              n121 = Build Array(w374, w373, w372) -> (w371:path[])
              n122 = for {
                tunnel: w371 -> [w381] mode=indexing
                tunnel: w370 -> [w382]
                tunnel: [w379] -> w369 mode=indexing
                n123 = for {
                  tunnel: w382 -> [w386] mode=indexing
                  tunnel: w381 -> [w384]
                  tunnel: [w383] -> w380 mode=indexing
                  n124 = Unbundle By Name(w386) -> ("ClassFolder"=w385:path)
                  n125 = Equal?(x=w385, y=w384) -> (x = y?=w383:bool)
                }
                n126 = Or Array Elements(Boolean array=w380) -> (logical OR=w379:bool)
              }
              n127 = Or Array Elements(Boolean array=w369) -> (logical OR=w368:bool)
              n128 = case shown="False" w368 {
                tunnel: [w376 w378] -> w367
                tunnel: w366 -> [w377 w378]
                tunnel: w365 -> [w375 _]
                frame False {
                  n129 = Build Array (concatenate)(w377, w375) -> (w376:path[])
                }
                frame True {
                }
              }
            }
          }
        }
        n130 = stacked-sequence {
          tunnel: w331 -> [w341]
          tunnel: w332 -> [w343]
          frame #0 {
            n131 = for {
              tunnel: w341 -> [w353] mode=indexing
              tunnel: [w350] -> w349 mode=indexing
              n132 = Unbundle By Name(w353) -> ("ClassName"=w352:string)
              n133 = Concatenate Strings(w352, "\n" ("string")) -> (w350:string)
            }
            n134 = Empty Array?(array=w341) -> (empty?=w344:bool)
            n135 = Array Size(array=w343) -> (size(s)=→"Additional VIs that has been found\nand will be relinked:":i32)
            n136 = Select(t=u8 2, s=w344, f=u8 0 ("Disabled")) -> (s? t:f=w347:u8)
            n137 = property on="Next" class="Bool"("Disabled"=w347) -> ()  [unwired: 2 in, 2 out]
            n138 = Concatenate Strings(w349) -> (→"GOOP1 classes found":string)
          }
        }
        n139 = Bundle By Name(cluster=w334, "VIsToRelink(Paths)"=w332) -> (w333:T7)
      }
      frame "CreateProject" {
        n140 = Open Application Reference(8:w397) -> (0:w398:errorcluster, 3:w396:refnum<vi>)  [unwired: 3 in]
        n141 = invoke class="App" method="Project.New"(reference=w396, error in=w398) -> (reference out=w387:refnum<vi>, error out=w400:errorcluster, "Project:New"=w403:refnum<vi>)  [unwired: 1 in]
        n142 = Unbundle By Name(w401) -> ("Project"=w402:path)
        n143 = invoke class="Project" method="Save"(reference=w403, error in=w400, "Path"=w402) -> (reference out=w392:refnum<vi>, error out=w393:errorcluster)  [unwired: 1 in, 2 out]
        n144 = property class="Project"(reference=w392, error in=w393) -> (reference out=w391:refnum<vi>, error out=w390:errorcluster, "App Ref"=w394:refnum<vi>)
        n145 = property class="Project"(reference=w391, error in=w390) -> (error out=w388:errorcluster, "My Computer"=w389:refnum<vi>)  [unwired: 1 out]
        n146 = Bundle By Name(cluster=w401, "ProjectRef"=w391, "AppRef"=w394, "My Computer"=w389) -> (w399:T7)
        n147 = Close Reference(reference=w387, error in (no error)=w388) -> ()  [unwired: 1 out]
      }
      frame "OpenVIsToRelink" {
        n148 = Unbundle By Name(w412) -> ("AppRef"=w410:refnum<vi>, "VIsToRelink(Paths)"=w404:path[])
        n149 = for {
          tunnel: w410 -> [w418]
          shift-right: [w416] -> w408
          shift-left: w409 -> [w417]
          tunnel: [w415] -> w407 mode=indexing
          tunnel: w404 -> [w413] mode=indexing
          n150 = Empty String/Path?(string/path=w413) -> ()  [unwired: 1 out]
          n151 = Open VI Reference(application reference (local)=w418, vi path=w413, options=2, error in (no error)=w417) -> (vi reference=w415:refnum<vi>, error out=w416:errorcluster)  [unwired: 2 in]
        }
        n152 = property on="Progress" class="LstBox (strict)"("Item Names"=string[] ["Loading VIs in memory"]) -> ()  [unwired: 2 in, 2 out]
        n153 = Bundle By Name(cluster=w412, "VIsToRelink"=w407) -> (w411:T7)
      }
      frame "OpenClassesInMemory" {
        n154 = Unbundle By Name(w428) -> ("AppRef"=w423:refnum<vi>, "Classes"=w429:T2[])
        n155 = for {
          tunnel: w429 -> [w436] mode=indexing
          tunnel: [w434] -> w424 mode=indexing
          tunnel: w426 -> [w433]
          tunnel: w423 -> [w430]
          n156 = Unbundle By Name(w436) -> ("ClassFolder"=w439:path)  [unwired: 1 out]
          n157 = call <vilib>:"Recursive File List.vi"("Folder Path"=w439) -> ("All Files in Dir"=w438:path[])  [unwired: 6 in, 4 out]
          n158 = for {
            tunnel: w438 -> [w447] mode=indexing
            shift-right: [w448] -> w435
            shift-left: refnum<vi>[] [] -> [w449]
            tunnel: w433 -> [w445]
            shift-right: [w443] -> w432
            shift-left: path[] [] -> [w444]
            tunnel: w430 -> [w441]
            n159 = Strip Path(path=w447) -> (name=w446:string)  [unwired: 1 out]
            n160 = for {
              tunnel: w446 -> [w453]
              tunnel: w445 -> [w452] mode=indexing
              tunnel: [w450] -> w442 mode=indexing
              n161 = Match Pattern(string=w453, regular expression=w452) -> (offset past match=w451:i32)  [unwired: 1 in, 3 out]
              n162 = Greater Or Equal To 0?(x=w451) -> (x >= 0?=w450:bool)
            }
            n163 = Or Array Elements(Boolean array=w442) -> (logical OR=w440:bool)
            n164 = case shown="False" w440 {
              tunnel: w447 -> [w454 w458]
              tunnel: w449 -> [w456 w462]
              tunnel: [w456 w461] -> w448
              tunnel: w444 -> [w455 w460]
              tunnel: [w455 w459] -> w443
              tunnel: w441 -> [_ w457]
              frame True {
                n165 = Delete(path (use dialog)=w454) -> ()  [unwired: 4 in, 3 out]
              }
              frame False {
                n166 = call <resource>:"Scripting_OpenViRef.vi"("ViPath/ViName/Viref"=w458, "AppRef"=w457) -> ("error out"=w464:errorcluster, "vi reference"=w463:refnum<vi>)  [unwired: 7 in, 1 out]
                n167 = case shown="Error" w464 {
                  tunnel: w463 -> [w470 _]
                  tunnel: w462 -> [w469 w472]
                  tunnel: [w468 w472] -> w461
                  tunnel: w460 -> [w467 w471]
                  tunnel: [w466 w471] -> w459
                  tunnel: w458 -> [w465 _]
                  frame No Error {
                    n168 = Build Array (concatenate)(w467, w465) -> (w466:path[])
                    n169 = Build Array (concatenate)(w469, w470) -> (w468:refnum<vi>[])
                  }
                  frame Error {
                  }
                }
              }
            }
          }
          n170 = Bundle By Name(cluster=w436, "ViRefs"=w435, "ViPathes"=w432) -> (w434:T2)
        }
        n171 = Bundle By Name(cluster=w428, "Classes"=w424) -> (w427:T7)
        n172 = property on="Progress" class="LstBox (strict)"() -> ("Item Names"=w422:string[])  [unwired: 2 in, 2 out]
        n173 = Build Array (concatenate)(w422, "Loading Class VIs in memory") -> (w421:string[])
        n174 = property on="Progress" class="LstBox (strict)"("Item Names"=w421) -> ()  [unwired: 2 in, 2 out]
      }
      frame "RemoveReentrantForDynamicDispatchVIs" {
        n175 = Unbundle By Name(w477) -> ("Classes"=w474:T2[])
        n176 = for {
          tunnel: w474 -> [w487] mode=indexing
          shift-right: [w485] -> w475
          shift-left: w476 -> [w486]
          tunnel: w474 -> [w482]
          i -> [w481]
          n177 = Delete From Array(array=w482, index=w481) -> (array with subset deleted=w480:T2[])  [unwired: 1 in, 1 out]
          n178 = Unbundle By Name(w487) -> ("ViRefs"=w484:refnum<vi>[], "ViPathes"=w483:path[])
          n179 = for {
            tunnel: w480 -> [w492] mode=indexing
            shift-right: [w490] -> w478
            shift-left: string[] [] -> [w491]
            n180 = Unbundle By Name(w492) -> ("ViPathes"=w488:path[])
            n181 = for {
              tunnel: [w494] -> w489 mode=indexing
              tunnel: w488 -> [w493] mode=indexing
              n182 = Strip Path(path=w493) -> (name=w494:string)  [unwired: 1 out]
            }
            n183 = Build Array (concatenate)(w491, w489) -> (w490:string[])
          }
          n184 = for {
            shift-right: [w507] -> w485
            shift-left: w486 -> [w508]
            tunnel: w484 -> [w506] mode=indexing
            tunnel: w483 -> [w505] mode=indexing
            tunnel: w478 -> [w498]
            n185 = Strip Path(path=w505) -> (stripped path=w504:path, name=w500:string)
            n186 = To Lower Case(string=w498) -> (all lower case string=w497:string[])
            n187 = To Lower Case(string=w500) -> (all lower case string=w499:string)
            n188 = Strip Path(path=w504) -> (name=w503:string)  [unwired: 1 out]
            n189 = Search 1D Array(1D array=w497, element=w499) -> (index of element=w496:i32)  [unwired: 1 in]
            n190 = Not Equal?(x=w503, y="utils") -> (x != y?=w501:bool)
            n191 = Greater Or Equal To 0?(x=w496) -> (x >= 0?=w495:bool)
            n192 = case shown="True" w501 {
              tunnel: w508 -> [w509 w510]
              tunnel: [w509 w510] -> w507
              tunnel: w506 -> [_ w512]
              tunnel: w495 -> [_ _]
              frame False {
              }
              frame True {
                n193 = property class="VI"(reference=w512, error in=w510, "Exec.IsReentrant"=FALSE ("Execution:Is Reentrant")) -> ()  [unwired: 2 out]
              }
            }
          }
        }
      }
      frame "RecompilingVIs" {
        n194 = Unbundle By Name(w513) -> ("Classes"=w515:T2[], "VIsToRelink"=w514:refnum<vi>[])
        n195 = call <resource>:"ConvertGoop2ToGoop3_RecompileAll.vi"("error IO 2"=w521, "VIsToRelink"=w514, "Classes"=w515) -> ("error IO"=w520:errorcluster)  [unwired: 6 in]
        n196 = property on="Progress" class="LstBox (strict)"() -> ("Item Names"=w518:string[])  [unwired: 2 in, 2 out]
        n197 = Build Array (concatenate)(w518, "Recompiling VIs") -> (w517:string[])
        n198 = property on="Progress" class="LstBox (strict)"("Item Names"=w517) -> ()  [unwired: 2 in, 2 out]
      }
      frame "AddVIsToProject" {
        n199 = Unbundle By Name(w524) -> ("ProjectRef"=w523:refnum<vi>, "My Computer"=w522:refnum<vi>)
        n200 = Unbundle By Name(w524) -> ("TopFolderPath"=w525:path, "VIsToRelink(Paths)"=w532:path[])
        n201 = for {
          tunnel: w532 -> [w534] mode=indexing
          shift-right: [w533] -> w527
          shift-left: w531 -> [w533]
          tunnel: w525 -> [w541]
          tunnel: w522 -> [w537]
          tunnel: w523 -> [w536]
          n202 = Strip Path(path=w534) -> (stripped path=w540:path, name=w535:string)
          n203 = call <vilib>:"Compare Two Paths.vi"("Path 2"=w540, "Path 1"=w541) -> ("Relative Path from 1 to 2"=w539:path)  [unwired: 6 in, 3 out]
          n204 = Path To String(path=w539) -> (string=w538:string)
          n205 = case shown="\"\", \".\"" w538 {
            selector: w538 -> [w555 _]
            tunnel: w537 -> [w554 w559]
            tunnel: w536 -> [w544 _]
            tunnel: w533 -> [w551 _]
            tunnel: w535 -> [w550 w560]
            tunnel: w534 -> [w549 w561]
            tunnel: [w545 w558] -> _
            frame Default {
              n206 = call <resource>:"GDSProject_CreateFolder.vi"("Project Refnum In"=w544, "Project Item To Create Folder Below(Use MyComputer if not wired)"=w554, "FolderName"=w555, "error in (no error)"=w551) -> ("ItemOut"=w543:refnum<vi>, "error out"=w552:errorcluster)  [unwired: 12 in, 2 out]
              n207 = invoke class="ProjectItem" method="AddItem"(reference=w543, error in=w552, "Name"=w550, "Path"=w549, "Type"="VI") -> (reference out=w547:refnum<vi>, error out=w548:errorcluster, "AddItem"=w542:refnum<vi>)  [unwired: 1 in, 3 out]
              n208 = Close Reference(reference=w547, error in (no error)=w548) -> (error out=w546:errorcluster)
              n209 = Close Reference(reference=w542, error in (no error)=w546) -> (error out=w545:errorcluster)
            }
            frame "", "." {
              n210 = invoke class="TargetItem" method="AddItem"(reference=w559, "Name"=w560, "Path"=w561, "Type"="VI") -> (error out=w556:errorcluster, "AddItem"=w557:refnum<vi>)  [unwired: 2 in, 4 out]
              n211 = Close Reference(reference=w557, error in (no error)=w556) -> (error out=w558:errorcluster)
            }
          }
        }
        n212 = property on="Progress" class="LstBox (strict)"() -> ("Item Names"=w530:string[])  [unwired: 2 in, 2 out]
        n213 = Build Array (concatenate)(w530, "Adding VIs to project") -> (w529:string[])
        n214 = property on="Progress" class="LstBox (strict)"("Item Names"=w529) -> ()  [unwired: 2 in, 2 out]
      }
      frame "RenameFiles" {
        n215 = Unbundle By Name(w566) -> ("My Computer"=w569:refnum<vi>, "TopFolderPath"=w574:path)
        n216 = Unbundle By Name(w566) -> ("Classes"=w575:T2[])
        n217 = for {
          tunnel: w575 -> [w602] mode=indexing
          tunnel: w574 -> [_]
          shift-right: [w588] -> w573
          shift-left: w572 -> [w580]
          tunnel: [w608] -> w570 mode=indexing
          tunnel: w569 -> [w587]
          shift-right: [w604] -> w568
          shift-left: path[] [] -> [w605]
          tunnel: w566 -> [w601]
          shift-right: [w579] -> w563
          shift-left: path[] [] -> [w578]
          n218 = Unbundle By Name(w602) -> ("ClassName"=w584:string, "ClassFolder"=w581:path, "ClassPrefix"=w609:string, "IsLLB"=w577:bool, "ViRefs"=w603:refnum<vi>[])
          n219 = Unbundle By Name(w602) -> ("ClassName"=w606:string)
          n220 = Format Into String(format string="Renaming class: %s", w606) -> (resulting string=w592:string)  [unwired: 2 in, 1 out]
          n221 = property on="Progress" class="LstBox (strict)"() -> ("Item Names"=w600:string[], "Number of Rows"=w594:u32)  [unwired: 2 in, 2 out]
          n222 = Build Array (concatenate)(w600, w592) -> (w595:string[])
          n223 = Array Size(array=w595) -> (size(s)=w599:i32)
          n224 = Subtract(x=w599, y=w594) -> (x-y=w598:u32)
          n225 = To Long Integer(number=w598) -> (32bit integer=w596:i32)
          n226 = Max & Min(x=w596, y=0) -> (max(x,y)=w593:i32)  [unwired: 1 out]
          n227 = property on="Progress" class="LstBox (strict)"("Item Names"=w595, "Top Row"=w593) -> (error out=w591:errorcluster)  [unwired: 2 in, 1 out]
          n228 = for {
            tunnel: w603 -> [w639] mode=indexing
            shift-right: [w616] -> _
            shift-left: w580 -> [w616]
            tunnel: w609 -> [w637]
            tunnel: [w634] -> w589 mode=indexing
            tunnel: w581 -> [w633]
            tunnel: [w632] -> w583
            shift-right: [w630] -> w604
            shift-left: w605 -> [w629]
            tunnel: [w626] -> w585 mode=indexing
            tunnel: w601 -> [w623]
            tunnel: w591 -> [_]
            tunnel: [w617] -> _
            n229 = property class="VI"(reference=w639, error in=w616) -> (reference out=w638:refnum<vi>, error out=w625:errorcluster, "Path"=w631:path, "OwningApp"=w622:refnum<vi>)
            n230 = while {
              shift-right: [w640] -> w618
              shift-left: _ -> [w642]
              stop <- TRUE stop-if-true
              n231 = Increment(x=w642) -> (x+1=w641:i32)
              n232 = To Long Integer(number=w641) -> (32bit integer=w640:i32)
            }
            n233 = disable-structure shown="Enabled" {
              disable-tunnel: w625 -> [w646 w647]
              disable-tunnel: [w645 w647] -> w624
              disable-tunnel: w623 -> [_ _]
              frame Disabled {
                n234 = call <resource>:"ConvertGoop2ToGoop3_RecompileAll.vi"("error IO 2"=w646) -> ("error IO"=w645:errorcluster)  [unwired: 8 in]
              }
              frame Enabled {
              }
            }
            n235 = Strip Path(path=w631) -> ()  [unwired: 2 out]
            n236 = property class="App"(reference=w622) -> (reference out=w614:refnum<vi>, error out=w615:errorcluster, "App.Name"=w621:string)  [unwired: 1 in]
            n237 = Format Into String(format string="TempName%d.", w618) -> (resulting string=w619:string)  [unwired: 2 in, 1 out]
            n238 = call <resource>:"ConvertGoop1ToGoop3_KeepViPrefix.vi"("OrgViName"=w631, "ClassFolder"=w633, "error in (no error)"=w624, "ClassPrefix"=w637) -> ("ClassFolderOut"=w632:path, "Don'tUseVI"=w627:bool, "NewClassPath"=w628:path, "NewClassPathWithPreFix"=w636:path, "error out"=w635:errorcluster)  [unwired: 10 in, 1 out]
            n239 = Close Reference(reference=w614, error in (no error)=w615) -> ()  [unwired: 1 out]
            n240 = case shown="False" w627 {
              tunnel: w638 -> [w667 w703]
              tunnel: w636 -> [w656 _]
              tunnel: w635 -> [w665 w700]
              tunnel: [w662 w698] -> w617
              tunnel: w628 -> [w653 _]
              tunnel: [w664 w699] -> w634
              tunnel: w631 -> [w661 w699]
              tunnel: w631 -> [_ w695]
              tunnel: [w660 w696] -> w630
              tunnel: w629 -> [w659 w697]
              tunnel: [w658 _] -> w626
              tunnel: w621 -> [w654 _]
              tunnel: w619 -> [w651 _]
              frame False {
                # "Remove\nPrefix ?"
                n241 = call <vilib>:"Get File Extension.vi"("file"=w653) -> ("filename without extension"=w652:string, "lowercase file extension"=w650:string)  [unwired: 6 in, 3 out]
                n242 = Strip Path(path=w656) -> (name=w655:string)  [unwired: 1 out]
                n243 = invoke class="VI" method="Save.Instrument"(reference=w667, error in=w665, "Path to saved file"=w653) -> (reference out=w658:refnum<vi>, error out=w666:errorcluster)  [unwired: 3 in, 4 out]
                n244 = Strip Path(path=w653) -> (stripped path=w649:path, name=w657:string)
                n245 = Concatenate Strings(w652, w651, w650) -> (w648:string)
                n246 = case shown="No Error" w666 {
                  selector: w666 -> [w673 _]
                  tunnel: [w673 w680] -> w662
                  tunnel: w656 -> [_ w681]
                  tunnel: w665 -> [_ w683]
                  tunnel: w658 -> [_ w682]
                  tunnel: [w672 w681] -> w664
                  tunnel: w653 -> [w672 _]
                  tunnel: w657 -> [_ w679]
                  tunnel: w655 -> [_ w678]
                  tunnel: w654 -> [_ w677]
                  tunnel: w649 -> [_ w676]
                  tunnel: w648 -> [_ w675]
                  frame No Error {
                    # "Prefix\nRemoved"
                  }
                  frame Error {
                    # "..not\npossible"
                    n247 = Build Path(base path=w676, name or relative path=w675) -> (appended path=w674:path)
                    n248 = stacked-sequence {
                      tunnel: w679 -> [w686]
                      tunnel: w678 -> [w685]
                      tunnel: [w685] -> _
                      tunnel: w677 -> [w684]
                      frame #0 {
                        w690 = path "c:/G2To3.txt" ("file (use dialog)")
                        n249 = Read from Text File(file (use dialog)=w690) -> (text=w687:string)  [unwired: 3 in, 3 out]
                        n250 = Format Into String(format string="       %s(%s)%s\n", initial string=w687, w686, w685, w684) -> (resulting string=w689:string)  [unwired: 1 in, 1 out]
                        n251 = stacked-sequence {
                          tunnel: w689 -> [w693]
                          tunnel: w690 -> [w691]
                          frame #0 {
                            n252 = Delete(path (use dialog)=w691) -> (deleted path=w692:path)  [unwired: 4 in, 2 out]
                            n253 = Write to Text File(file (use dialog)=w692, text=w693) -> ()  [unwired: 2 in, 3 out]
                          }
                        }
                      }
                    }
                    n254 = invoke class="VI" method="Save.Instrument"(reference=w682, error in=w683, "Path to saved file"=w674) -> (error out=w680:errorcluster)  [unwired: 3 in, 5 out]
                  }
                }
                n255 = Not Equal?(x=w664, y=w661) -> (x != y?=w663:bool)
                n256 = case shown="True" w663 {
                  tunnel: w662 -> [_ _]
                  tunnel: w661 -> [_ w669]
                  tunnel: [w668 w671] -> w660
                  tunnel: w659 -> [w668 w670]
                  frame False {
                  }
                  frame True {
                    n257 = Build Array (concatenate)(w670, w669) -> (w671:path[])
                  }
                }
              }
              frame True {
                n258 = case shown="False" FALSE {
                  tunnel: w703 -> [w705 w709]
                  tunnel: [w705 w708] -> w702
                  tunnel: [w704 w707] -> w701
                  tunnel: w700 -> [w704 w706]
                  frame False {
                  }
                  frame True {
                    n259 = invoke class="VI" method="Save.Instrument"(reference=w709, error in=w706) -> (reference out=w708:refnum<vi>, error out=w707:errorcluster)  [unwired: 4 in, 4 out]
                  }
                }
                n260 = Close Reference(reference=w702, error in (no error)=w701) -> (error out=w698:errorcluster)
                n261 = Build Array (concatenate)(w697, w695) -> (w696:path[])
              }
            }
            n262 = stacked-sequence {
              tunnel: w617 -> [_]
              frame #0 {
                n263 = Wait (ms)(milliseconds to wait=u32 2) -> ()  [unwired: 1 out]
              }
            }
          }
          n264 = case shown="False" w577 {
            tunnel: w581 -> [_ w611]
            tunnel: [w610 w613] -> w579
            tunnel: w578 -> [w610 w612]
            frame False {
            }
            frame True {
              n265 = Build Array (concatenate)(w612, w611) -> (w613:path[])
            }
          }
          n266 = call <resource>:"ConvertGoop2ToGoop3_CreateLvClass.vi"("ClassFolder"=w583, "ProjectItem"=w587, "ClassName"=w584, "ViRefsIn"=w585, "ViPathsIn"=w589, "error in"=w580) -> ("LvClassCreated"=w582:refnum<vi>, "ViRefsOut"=w586:refnum<vi>[], "ViPathsOut"=w590:path[], "error out"=w588:errorcluster)  [unwired: 6 in]
          n267 = Bundle By Name(cluster=w602, "ClassFolder"=w583, "ViRefs"=w586, "ViPathes"=w590, "ClassRef"=w582) -> (w608:T2)
        }
        n268 = Bundle By Name(cluster=w566, "LLBsToDelete"=w563, "Classes"=w570) -> (w571:T7)
        n269 = for {
          tunnel: w568 -> [w576] mode=indexing
          n270 = Delete(path (use dialog)=w576) -> ()  [unwired: 4 in, 3 out]
        }
      }
      frame "RenameTempNames" {
        n271 = Unbundle By Name(w711) -> ("Classes"=w714:T2[])
        n272 = for {
          tunnel: w714 -> [w716] mode=indexing
          shift-right: [w715] -> w713
          shift-left: w712 -> [w719]
          tunnel: w711 -> [w717]
          n273 = Unbundle By Name(w716) -> ("ViRefs"=w718:refnum<vi>[])
          n274 = for {
            tunnel: w718 -> [w725] mode=indexing
            shift-right: [w722] -> w715
            shift-left: w719 -> [w720]
            tunnel: w717 -> [_]
            n275 = property class="VI"(reference=w725, error in=w720) -> (reference out=w723:refnum<vi>, error out=w721:errorcluster, "Path"=w724:path)
            n276 = case shown="No Error" w721 {
              selector: w721 -> [w726 _]
              tunnel: w724 -> [w730 _]
              tunnel: w723 -> [w729 _]
              tunnel: [w728 w745] -> w722
              tunnel: w720 -> [_ w745]
              frame No Error {
                n277 = call <vilib>:"Get File Extension.vi"("file"=w730) -> ("filename without extension"=w734:string)  [unwired: 6 in, 4 out]
                n278 = Match Pattern(string=w734, regular expression="TempName[0-9]+") -> (before substring=w732:string, after substring=w731:string, offset past match=w727:i32)  [unwired: 1 in, 1 out]
                n279 = case shown="-1" w727 {
                  tunnel: w732 -> [w743 _]
                  tunnel: w731 -> [w742 _]
                  tunnel: w730 -> [w741 _]
                  tunnel: w729 -> [w738 _]
                  tunnel: w726 -> [w737 w744]
                  tunnel: [w736 w744] -> w728
                  frame 0, Default {
                    n280 = Concatenate Strings(w743, w742) -> (w739:string)
                    n281 = Strip Path(path=w741) -> (stripped path=w740:path)  [unwired: 1 out]
                    n282 = Build Path(base path=w740, name or relative path=w739) -> (appended path=w735:path)
                    n283 = invoke class="VI" method="Save.Instrument"(reference=w738, error in=w737, "Path to saved file"=w735) -> (error out=w736:errorcluster)  [unwired: 3 in, 5 out]
                  }
                  frame -1 {
                  }
                }
              }
              frame Error {
              }
            }
          }
        }
      }
      frame "CreateCopyClasses" {
        n284 = Open Application Reference(8:w773) -> (0:w779:errorcluster, 3:w778:refnum<vi>)  [unwired: 3 in]
        n285 = Temporary Directory() -> (w772:path)
        n286 = invoke class="App" method="Project.New"(reference=w778, error in=w779) -> (reference out=w748:refnum<vi>, error out=w757:errorcluster, "Project:New"=w780:refnum<vi>)  [unwired: 1 in]
        n287 = Unbundle By Name(w754) -> ("Classes"=w767:T2[])
        n288 = Build Path(base path=w772, name or relative path="G12G3_folder") -> (appended path=w770:path)
        n289 = Delete(path (use dialog)=w770, entire hierarchy (F)=TRUE) -> (deleted path=w766:path)  [unwired: 3 in, 2 out]
        n290 = Create Folder(path (use dialog)=w766, error in=w757) -> (created path=w752:path, error out=w756:errorcluster)  [unwired: 1 in, 1 out]
        n291 = Build Path(base path=w752, name or relative path="G12G3_Temp.lvproj") -> (appended path=w762:path)
        n292 = invoke class="Project" method="Save"(reference=w780, error in=w756, "Path"=w762) -> (reference out=w776:refnum<vi>, error out=w777:errorcluster)  [unwired: 1 in, 2 out]
        n293 = property class="Project" props=["App Ref"](reference=w776, error in=w777) -> (reference out=w775:refnum<vi>, error out=w774:errorcluster)  [unwired: 1 out]
        n294 = property class="Project"(reference=w775, error in=w774) -> (reference out=w759:refnum<vi>, error out=w765:errorcluster, "My Computer"=w760:refnum<vi>)
        n295 = Format Into String(EndevoTemplateNames."BaseTemplate" ("TemplateNames")) -> (resulting string=w763:string)  [unwired: 3 in, 1 out]
        n296 = for {
          tunnel: T10 {"ClassName"="", "ClassFolder"=path "", "ClassDescription"="", "ClassTemplateOptions"="", "BaseClass(ProjectStringPath or LvClassFilePath)"=variant, "ExtraCreateParameters"=variant, "FolderSuffix"=""} ("CreateClassData") -> [w806]
          tunnel: w760 -> [w804]
          tunnel: w767 -> [w803] mode=indexing
          shift-right: [w799] -> w761
          shift-left: w765 -> [w800]
          tunnel: w752 -> [w794]
          tunnel: w763 -> [w793]
          tunnel: [w781] -> w746 mode=indexing
          n297 = Unbundle By Name(w803) -> ("ClassName"=w782:string, "ClassFolder"=w796:path, "ViRefs"=w802:refnum<vi>[])
          n298 = Index Array(array=w802) -> (element=w801:refnum<vi>)  [unwired: 1 in]
          n299 = Strip Path(path=w796) -> (name=w797:string)  [unwired: 1 out]
          n300 = Build Path(base path=w794, name or relative path=w797) -> (appended path=w795:path)
          n301 = Bundle By Name(cluster=w806, "ClassName"=w782, "ClassFolder"=w795, "ClassTemplateOptions"=w793) -> (w805:T10)
          n302 = Format Into String(format string="Creating Copy Class: %s", w782) -> (resulting string=w783:string)  [unwired: 2 in, 1 out]
          n303 = property on="Progress" class="LstBox (strict)"() -> ("Item Names"=w792:string[], "Number of Rows"=w786:u32)  [unwired: 2 in, 2 out]
          n304 = Build Array (concatenate)(w792, w783) -> (w787:string[])
          n305 = Array Size(array=w787) -> (size(s)=w791:i32)
          n306 = Subtract(x=w791, y=w786) -> (x-y=w790:u32)
          n307 = To Long Integer(number=w790) -> (32bit integer=w788:i32)
          n308 = Max & Min(x=w788, y=0) -> (max(x,y)=w785:i32)  [unwired: 1 out]
          n309 = property on="Progress" class="LstBox (strict)"("Item Names"=w787, "Top Row"=w785) -> ()  [unwired: 2 in, 2 out]
          n310 = call-dynamic "CreateClass.vi"("ClassWriterGOOP300.lvclass"=refnum<class "ClassWriterGOOP300.lvclass"> refnum, "ProjectTreePosition(String or Project Item Ref)"=w804, "CreateClassData"=w805, "error in (no error)"=w800, "KeepLvClassRefOpen(False)"=FALSE, "HeaderToApply (take from VIRef or /use 2D-8bit header, Ignored if not wired)"=w801) -> ("TemplateVersionUsed"=w781:string, "error out"=w799:errorcluster)  [unwired: 10 in, 2 out]
        }
        n311 = invoke class="Project" method="Save"(reference=w759, error in=w761) -> (reference out=w750:refnum<vi>, error out=w751:errorcluster)  [unwired: 2 in, 2 out]
        n312 = Bundle By Name(cluster=w754, "CopyClasses"=w752, "TemplateVersions"=w746) -> (w753:T7)
        n313 = Close Reference(reference=w750, error in (no error)=w751) -> (error out=w749:errorcluster)
        n314 = Close Reference(reference=w760, error in (no error)=w761) -> ()  [unwired: 1 out]
        n315 = Close Reference(reference=w748, error in (no error)=w749) -> (error out=w747:errorcluster)
      }
      frame "UpdateVIsGoopRefs" {
        (unwired) "UpdateCreate"
        n316 = Unbundle By Name(w812) -> ("Classes"=w817:T2[])
        n317 = for {
          tunnel: w817 -> [w831] mode=indexing
          tunnel: [w829] -> w814 mode=indexing
          n318 = Unbundle By Name(w831) -> ("ClassRef"=w830:refnum<vi>)
          n319 = property class="LVClassLibrary"(reference=w830) -> ("Path"=w829:path)  [unwired: 1 in, 2 out]
        }
        n320 = for {
          tunnel: w817 -> [w848] mode=indexing
          shift-right: [w832] -> w816
          shift-left: w818 -> [w847]
          tunnel: w814 -> [w845]
          n321 = Unbundle By Name(w848) -> ("ViRefs"=w846:refnum<vi>[], "ViPathes"=w844:path[], "ClassName"=w834:string)  [unwired: 2 out]
          n322 = for {
            shift-right: [w861] -> w832
            shift-left: w847 -> [w862]
            tunnel: w846 -> [w852] mode=indexing
            tunnel: w845 -> [w860]
            tunnel: w844 -> [w854] mode=indexing
            tunnel: [w853] -> _
            n323 = Strip Path(path=w854) -> (stripped path=w859:path, name=w856:string)
            n324 = Path To String(path=w854) -> (string=w853:string)
            n325 = Match Pattern(string=w856, regular expression="\\2E[Vv][Ii]$") -> ()  [unwired: 1 in, 4 out]
            n326 = Strip Path(path=w859) -> (name=w858:string)  [unwired: 1 out]
            n327 = Not Equal?(x=w858, y="utils") -> ()  [unwired: 1 out]
            n328 = Not A Number/Path/Refnum?(number/path/refnum=w852) -> (NaN/Path/Refnum?=w851:bool)
            n329 = Compound Arithmetic op=AND(invert w851) -> (w850:bool)
            n330 = case shown="True" w850 {
              tunnel: w862 -> [w863 w864]
              tunnel: [w863 w864] -> w861
              tunnel: w852 -> [_ w866]
              tunnel: w860 -> [_ w865]
              frame False {
              }
              frame True {
                n331 = call <resource>:"Scripting_ReplaceGoop2OORef.vi"("ViRef"=w866, "Classes(.lvclass files)"=w865, "error in (no error)"=w864) -> ()  [unwired: 16 in, 1 out]
              }
            }
          }
          n332 = Format Into String(format string="Updating GOOP Ref: %s", w834) -> (resulting string=w833:string)  [unwired: 2 in, 1 out]
          n333 = property on="Progress" class="LstBox (strict)"() -> ("Item Names"=w843:string[], "Number of Rows"=w837:u32)  [unwired: 2 in, 2 out]
          n334 = Build Array (concatenate)(w843, w833) -> (w838:string[])
          n335 = Array Size(array=w838) -> (size(s)=w842:i32)
          n336 = Subtract(x=w842, y=w837) -> (x-y=w841:u32)
          n337 = To Long Integer(number=w841) -> (32bit integer=w839:i32)
          n338 = Max & Min(x=w839, y=0) -> (max(x,y)=w836:i32)  [unwired: 1 out]
          n339 = property on="Progress" class="LstBox (strict)"("Item Names"=w838, "Top Row"=w836) -> ()  [unwired: 2 in, 2 out]
          n340 = stacked-sequence {
            tunnel: w832 -> [_]
            frame #0 {
              n341 = Wait (ms)(milliseconds to wait=u32 5) -> ()  [unwired: 1 out]
            }
          }
        }
        n342 = Unbundle By Name(w812) -> ("VIsToRelink"=w815:refnum<vi>[])
        n343 = for {
          shift-right: [w819] -> w811
          shift-left: w816 -> [w823]
          tunnel: w815 -> [w822] mode=indexing
          tunnel: w814 -> [w820]
          n344 = Not A Number/Path/Refnum?(number/path/refnum=w822) -> (NaN/Path/Refnum?=w821:bool)
          n345 = case shown="False" w821 {
            tunnel: w823 -> [w827 w828]
            tunnel: [w827 w828] -> w819
            tunnel: w822 -> [w826 _]
            tunnel: w820 -> [w825 _]
            frame False {
              n346 = call <resource>:"Scripting_ReplaceGoop2OORef.vi"("ViRef"=w826, "Classes(.lvclass files)"=w825, "error in (no error)"=w827) -> ()  [unwired: 16 in, 1 out]
            }
            frame True {
            }
          }
          n347 = stacked-sequence {
            tunnel: w819 -> [_]
            frame #0 {
              n348 = Wait (ms)(milliseconds to wait=u32 5) -> ()  [unwired: 1 out]
            }
          }
        }
        n349 = Unbundle By Name(w812) -> ("Classes"=w809:T2[], "VIsToRelink"=w808:refnum<vi>[])
        n350 = call <resource>:"ConvertGoop2ToGoop3_RecompileAll.vi"("error IO 2"=w811, "VIsToRelink"=w808, "Classes"=w809) -> ("error IO"=w810:errorcluster)  [unwired: 6 in]
      }
      frame "CopyVIsOver" {
        n351 = Unbundle By Name(w869) -> ("CopyClasses"=w873:path, "Classes"=w870:T2[])
        n352 = for {
          tunnel: w870 -> [w941] mode=indexing
          tunnel: w873 -> [w939]
          shift-right: [w929] -> w871
          shift-left: w872 -> [w929]
          tunnel: [w928] -> _ mode=indexing
          tunnel: [w927] -> _ mode=indexing
          w931 = "protected" ("name or relative path")
          n353 = Unbundle By Name(w941) -> ("ClassFolder"=w926:path)  [unwired: 1 out]
          n354 = Strip Path(path=w926) -> (name=w925:string)  [unwired: 1 out]
          n355 = Build Path(base path=w939, name or relative path=w925) -> (appended path=w936:path)
          n356 = Build Path(base path=w926, name or relative path=w931) -> (appended path=w930:path)
          n357 = Build Path(base path=w936, name or relative path="utils") -> (appended path=w937:path)
          n358 = Build Path(base path=w936, name or relative path=w931) -> (appended path=w935:path)
          n359 = Build Path(base path=w935, name or relative path="ClassAttributes.ctl") -> (appended path=w933:path)
          n360 = Copy(9:TRUE ("overwrite (F)"), 10:w926, 11:w937) -> (0:w928:errorcluster)  [unwired: 2 in, 2 out]
          n361 = Copy(9:TRUE ("overwrite (F)"), 10:w930, 11:w933) -> (0:w927:errorcluster)  [unwired: 2 in, 2 out]
        }
        n362 = disable-structure shown="Enabled" {
          disable-tunnel: w871 -> [w883 w895]
          disable-tunnel: w870 -> [w882 w894]
          disable-tunnel: w869 -> [w881 _]
          disable-tunnel: [w874 w893] -> w868
          frame Disabled {
            n363 = for {
              tunnel: w882 -> [w889] mode=indexing
              shift-right: [w884] -> w875
              shift-left: w883 -> [w885]
              n364 = Unbundle By Name(w889) -> ("ClassRef"=w886:refnum<vi>, "ViRefs"=w888:refnum<vi>[])
              n365 = for {
                tunnel: w888 -> [w892] mode=indexing
                shift-right: [w890] -> w887
                shift-left: w885 -> [w891]
                n366 = Close Reference(reference=w892, error in (no error)=w891) -> (error out=w890:errorcluster)
              }
              n367 = Close Reference(reference=w886, error in (no error)=w887) -> (error out=w884:errorcluster)
            }
            n368 = Unbundle By Name(w881) -> ("AppRef"=w878:refnum<vi>, "ProjectRef"=w879:refnum<vi>, "My Computer"=w880:refnum<vi>)
            n369 = Close Reference(reference=w880, error in (no error)=w875) -> (error out=w877:errorcluster)
            n370 = Close Reference(reference=w879, error in (no error)=w877) -> (error out=w876:errorcluster)
            n371 = Close Reference(reference=w878, error in (no error)=w876) -> (error out=w874:errorcluster)
          }
          frame Enabled {
            n372 = for {
              tunnel: w894 -> [w911] mode=indexing
              shift-right: [w907] -> w893
              shift-left: w895 -> [w908]
              n373 = Unbundle By Name(w911) -> ("ViRefs"=w910:refnum<vi>[], "ViPathes"=w909:path[], "ClassName"=w896:string)
              n374 = for {
                tunnel: w910 -> [w913] mode=indexing
                tunnel: w909 -> [w920] mode=indexing
                shift-right: [w914] -> w907
                shift-left: w908 -> [w915]
                n375 = Strip Path(path=w920) -> (stripped path=w919:path)  [unwired: 1 out]
                n376 = property class="VI"(reference=w913) -> ("Path"=w912:path)  [unwired: 1 in, 2 out]
                n377 = Strip Path(path=w919) -> (name=w918:string)  [unwired: 1 out]
                n378 = Equal?(x=w918, y="utils" ("name or relative path")) -> (x = y?=w916:bool)
                n379 = case shown="True" w916 {
                  tunnel: w913 -> [_ w924]
                  tunnel: w915 -> [w921 w923]
                  tunnel: [w921 w922] -> w914
                  tunnel: w912 -> [_ _]
                  frame False {
                  }
                  frame True {
                    n380 = invoke class="VI" method="Revert VI"(reference=w924, error in=w923) -> (error out=w922:errorcluster)  [unwired: 1 in, 2 out]
                  }
                }
              }
              n381 = Format Into String(format string="Revert Class VIs: %s", w896) -> (resulting string=w897:string)  [unwired: 2 in, 1 out]
              n382 = property on="Progress" class="LstBox (strict)"() -> ("Item Names"=w906:string[], "Number of Rows"=w900:u32)  [unwired: 2 in, 2 out]
              n383 = Build Array (concatenate)(w906, w897) -> (w901:string[])
              n384 = Array Size(array=w901) -> (size(s)=w905:i32)
              n385 = Subtract(x=w905, y=w900) -> (x-y=w904:u32)
              n386 = To Long Integer(number=w904) -> (32bit integer=w902:i32)
              n387 = Max & Min(x=w902, y=0) -> (max(x,y)=w899:i32)  [unwired: 1 out]
              n388 = property on="Progress" class="LstBox (strict)"("Item Names"=w901, "Top Row"=w899) -> ()  [unwired: 2 in, 2 out]
            }
          }
        }
      }
      frame "RelinkAllSubVIs" {
        (unwired) "UpdateNewVI"
        n389 = Unbundle By Name(w944) -> ("Classes"=w945:T2[])
        n390 = for {
          tunnel: w945 -> [w962] mode=indexing
          shift-right: [w947] -> w943
          shift-left: w946 -> [w961]
          n391 = Unbundle By Name(w962) -> ("ViRefs"=w960:refnum<vi>[], "ViPathes"=w959:path[], "ClassName"=w949:string)  [unwired: 2 out]
          n392 = for {
            shift-right: [w974] -> w947
            shift-left: w961 -> [w975]
            tunnel: w960 -> [w966] mode=indexing
            tunnel: w959 -> [w968] mode=indexing
            tunnel: [w967] -> _
            n393 = Strip Path(path=w968) -> (stripped path=w973:path, name=w970:string)
            n394 = Path To String(path=w968) -> (string=w967:string)
            n395 = Match Pattern(string=w970, regular expression="\\2E[Vv][Ii]$") -> ()  [unwired: 1 in, 4 out]
            n396 = Strip Path(path=w973) -> (name=w972:string)  [unwired: 1 out]
            n397 = Equal?(x=w972, y="utils") -> ()  [unwired: 1 out]
            n398 = Not A Number/Path/Refnum?(number/path/refnum=w966) -> (NaN/Path/Refnum?=w965:bool)
            n399 = Compound Arithmetic op=AND(invert w965) -> (w964:bool)
            n400 = case shown="True" w964 {
              tunnel: w975 -> [w976 w977]
              tunnel: [w976 w977] -> w974
              tunnel: w966 -> [_ w979]
              frame False {
              }
              frame True {
                n401 = call <resource>:"Scripting_FindNodeOnDiagram.vi"("ViRef(Ignored If Not Wired)"=w979, "NodeTypesToSearchFor"=string[] ["SubVI"], "error in (no error)"=w977) -> ("Nodes"=w978:refnum<vi>[])  [unwired: 15 in, 1 out]
                n402 = for {
                  tunnel: w978 -> [w985] mode=indexing
                  w984 = refnum<vi> refnum  # SubVI
                  n403 = To More Specific Class(target class=w984, reference=w985) -> (specific class reference=w982:refnum<vi>, error out=w983:errorcluster)  [unwired: 1 in]
                  n404 = invoke class="SubVI" method="Relink To VI"(reference=w982, error in=w983) -> ("Relink To VI"=w981:refnum<vi>)  [unwired: 1 in, 2 out]
                  n405 = Close Reference(reference=w981) -> ()  [unwired: 1 in, 1 out]
                }
              }
            }
          }
          n406 = Format Into String(format string="Relink SubVIs in: %s", w949) -> (resulting string=w948:string)  [unwired: 2 in, 1 out]
          n407 = property on="Progress" class="LstBox (strict)"() -> ("Item Names"=w958:string[], "Number of Rows"=w952:u32)  [unwired: 2 in, 2 out]
          n408 = Build Array (concatenate)(w958, w948) -> (w953:string[])
          n409 = Array Size(array=w953) -> (size(s)=w957:i32)
          n410 = Subtract(x=w957, y=w952) -> (x-y=w956:u32)
          n411 = To Long Integer(number=w956) -> (32bit integer=w954:i32)
          n412 = Max & Min(x=w954, y=0) -> (max(x,y)=w951:i32)  [unwired: 1 out]
          n413 = property on="Progress" class="LstBox (strict)"("Item Names"=w953, "Top Row"=w951) -> ()  [unwired: 2 in, 2 out]
          n414 = stacked-sequence {
            tunnel: w947 -> [_]
            frame #0 {
              n415 = Wait (ms)(milliseconds to wait=u32 5) -> ()  [unwired: 1 out]
            }
          }
        }
      }
      frame "ConnectVIsToClass" {
        n416 = Unbundle By Name(w987) -> ("Classes"=w990:T2[])
        n417 = Unbundle By Name(w987) -> ("AppRef"=w986:refnum<vi>)
        n418 = for {
          tunnel: w990 -> [w1016] mode=indexing
          shift-right: [w1005] -> w988
          shift-left: w989 -> [w1006]
          tunnel: w986 -> [w992]
          n419 = Unbundle By Name(w1016) -> ("ClassRef"=w1002:refnum<vi>, "ClassFolder"=w995:path, "ViPathes"=w1007:path[], "ClassName"=w1010:string)  [unwired: 1 out]
          n420 = To More Generic Class(target class=refnum<vi> refnum ("AddItem"), reference=w1002) -> (generic class reference=w1003:refnum<vi>)
          n421 = call <vilib>:"Recursive File List.vi"("pattern"="*.vi", "Folder Path"=w995) -> ("All Files in Dir"=w1008:path[])  [unwired: 5 in, 4 out]
          n422 = call <vilib>:"Recursive File List.vi"("pattern"="*.ctl", "Folder Path"=w995) -> ("All Files in Dir"=w993:path[])  [unwired: 5 in, 4 out]
          n423 = Build Array (concatenate)(w1008, w993) -> (w994:path[])
          n424 = for {
            tunnel: w994 -> [w1021] mode=indexing
            tunnel: w1007 -> [w1026]
            shift-right: [w1023] -> w1005
            shift-left: w1006 -> [w1024]
            tunnel: w1003 -> [w1022]
            tunnel: w995 -> [w1020]
            tunnel: w1002 -> [w1019]
            tunnel: w1002 -> [w1018]
            tunnel: w992 -> [w1017]
            n425 = Search 1D Array(1D array=w1026, element=w1021) -> (index of element=w1025:i32)  [unwired: 1 in]
            n426 = case shown="-1" w1025 {
              tunnel: w1024 -> [w1027 w1062]
              tunnel: [w1027 w1068] -> w1023
              tunnel: w1022 -> [_ w1058]
              tunnel: w1021 -> [_ w1036]
              tunnel: w1020 -> [_ w1064]
              tunnel: w1019 -> [_ w1057]
              tunnel: w1018 -> [_ w1038]
              tunnel: w1017 -> [_ w1033]
              frame 0, Default {
              }
              frame -1 {
                (unwired) T11."private" ("Scope")
                n427 = call <vilib>:"Compare Two Paths.vi"("error in (no error)"=w1062, "Path 2"=w1036, "Path 1"=w1064) -> ("error out"=w1059:errorcluster, "Relative Path from 1 to 2"=w1063:path)  [unwired: 5 in, 2 out]
                n428 = Strip Path(path=w1063) -> (stripped path=w1061:path, name=w1040:string)
                n429 = Strip Path(path=w1036) -> (stripped path=w1066:path, name=w1067:string)
                n430 = Strip Path(path=w1061) -> (name=w1060:string)  [unwired: 1 out]
                n431 = case shown="Default" w1060 {
                  selector: w1060 -> [w1076 _]
                  tunnel: w1058 -> [w1082 w1101]
                  tunnel: [w1079 w1101] -> w1056
                  tunnel: w1059 -> [w1081 w1100]
                  tunnel: [w1077 w1100] -> w1034
                  tunnel: w1057 -> [w1080 _]
                  tunnel: [TRUE _] -> w1051
                  frame Default {
                    (unwired) "Folder"
                    n432 = call <resource>:"GDSProject_CreateFolder.vi"("Project Item To Create Folder Below(Use MyComputer if not wired)"=w1082, "FolderName"=w1076, "error in (no error)"=w1081) -> ("ItemOut"=w1079:refnum<vi>, "FolderCreated"=w1074:bool, "error out"=w1078:errorcluster)  [unwired: 13 in, 1 out]
                    n433 = case shown="True" w1074 {
                      tunnel: w1080 -> [_ w1088]
                      tunnel: w1079 -> [_ w1087]
                      tunnel: w1078 -> [w1083 w1086]
                      tunnel: [w1083 w1085] -> w1077
                      tunnel: w1076 -> [_ w1084]
                      frame False {
                      }
                      frame True {
                        n434 = case shown="Default" w1084 {
                          tunnel: w1088 -> [_ w1094 w1099]
                          tunnel: w1087 -> [_ w1093 w1098]
                          tunnel: w1086 -> [w1089 w1092 w1097]
                          tunnel: [w1089 w1091 w1096] -> w1085
                          frame "Public", "util", "utils" {
                          }
                          frame "protected" {
                            n435 = invoke class="LVClassLibrary" method="Set Source Scope"(reference=w1094, error in=w1092, "SourceRef"=w1093, "Scope"=T11."protected" ("scope")) -> (error out=w1091:errorcluster)  [unwired: 1 in, 4 out]
                          }
                          frame Default {
                            n436 = invoke class="LVClassLibrary" method="Set Source Scope"(reference=w1099, error in=w1097, "SourceRef"=w1098, "Scope"=T11."private" ("scope")) -> (error out=w1096:errorcluster)  [unwired: 1 in, 4 out]
                          }
                        }
                      }
                    }
                  }
                  frame "" {
                  }
                }
                n437 = call <resource>:"Scripting_OpenViRef.vi"("error in"=w1034, "ViPath/ViName/Viref"=w1036, "AppRef"=w1033) -> ("error out"=w1035:errorcluster, "vi reference"=w1032:refnum<vi>)  [unwired: 6 in, 1 out]
                n438 = Strip Path(path=w1066) -> (name=w1065:string)  [unwired: 1 out]
                n439 = invoke class="ProjectItem" method="AddItem"(reference=w1056, error in=w1035, "Name"=w1067, "Path"=w1036, "Type"="VI") -> (reference out=w1055:refnum<vi>, error out=w1029:errorcluster, "AddItem"=w1037:refnum<vi>)  [unwired: 1 in, 3 out]
                n440 = Match Pattern(string=w1040, regular expression="ObjectStatus") -> (offset past match=w1049:i32)  [unwired: 1 in, 3 out]
                n441 = Match Pattern(string=w1040, regular expression="GOOPKernel") -> (offset past match=w1045:i32)  [unwired: 1 in, 3 out]
                n442 = invoke class="VI" method="Save.Instrument"(reference=w1032, error in=w1029) -> (reference out=w1031:refnum<vi>, error out=w1030:errorcluster)  [unwired: 4 in, 4 out]
                n443 = Greater Or Equal To 0?(x=w1049) -> (x >= 0?=w1048:bool)
                n444 = Greater Or Equal To 0?(x=w1045) -> (x >= 0?=w1044:bool)
                n445 = Close Reference(reference=w1031, error in (no error)=w1030) -> (error out=w1028:errorcluster)
                n446 = Select(t=T11."protected" ("scope"), s=w1044, f=T11."private" ("scope")) -> (s? t:f=w1043:T11)
                n447 = Select(t=T11."public" ("scope"), s=w1048, f=w1043) -> (s? t:f=w1039:T11)
                n448 = case shown="\"False\", Default" w1065 {
                  tunnel: w1037 -> [w1102 w1104]
                  tunnel: w1028 -> [w1103 w1108]
                  tunnel: [w1103 w1107] -> w1054
                  tunnel: [w1102 w1104] -> w1052
                  tunnel: w1039 -> [_ w1106]
                  tunnel: w1038 -> [_ w1105]
                  frame "False", Default {
                  }
                  frame "util", "Utils" {
                    n449 = invoke class="LVClassLibrary" method="Set Source Scope"(reference=w1105, error in=w1108, "SourceRef"=w1104, "Scope"=w1106) -> (error out=w1107:errorcluster)  [unwired: 1 in, 4 out]
                  }
                }
                n450 = Close Reference(reference=w1052, error in (no error)=w1054) -> (error out=w1053:errorcluster)
                n451 = case shown="True" w1051 {
                  tunnel: [w1070 w1073] -> w1068
                  tunnel: w1055 -> [_ w1072]
                  tunnel: w1053 -> [w1070 w1071]
                  frame False {
                  }
                  frame True {
                    n452 = Close Reference(reference=w1072, error in (no error)=w1071) -> (error out=w1073:errorcluster)
                  }
                }
              }
            }
          }
          n453 = Format Into String(format string="Connecting VIs to class: %s", w1010) -> (resulting string=w1009:string)  [unwired: 2 in, 1 out]
          n454 = property on="Progress" class="LstBox (strict)"() -> ("Item Names"=w1000:string[], "Number of Rows"=w1001:u32)  [unwired: 2 in, 2 out]
          n455 = Build Array (concatenate)(w1000, w1009) -> (w999:string[])
          n456 = Array Size(array=w999) -> (size(s)=w1015:i32)
          n457 = Subtract(x=w1015, y=w1001) -> (x-y=w1014:u32)
          n458 = To Long Integer(number=w1014) -> (32bit integer=w1012:i32)
          n459 = Max & Min(x=w1012, y=0) -> (max(x,y)=w998:i32)  [unwired: 1 out]
          n460 = property on="Progress" class="LstBox (strict)"("Item Names"=w999, "Top Row"=w998) -> ()  [unwired: 2 in, 2 out]
        }
      }
      frame "UpdateLvClassIcon" {
        n461 = Unbundle By Name(w1111) -> ("Classes"=w1112:T2[], "AppRef"=w1124:refnum<vi>)
        n462 = for {
          tunnel: w1112 -> [w1169] mode=indexing
          shift-right: [w1128] -> w1114
          shift-left: w1126 -> [w1143]
          tunnel: w1124 -> [w1135]
          n463 = Unbundle By Name(w1169) -> ("ClassRef"=w1136:refnum<vi>, "ClassFolder"=w1158:path)
          n464 = List Folder(path=w1158, pattern="*.vi") -> (filenames=w1160:string[])  [unwired: 2 in, 3 out]
          n465 = Index Array(array=w1160) -> (element=w1159:string)  [unwired: 1 in]
          n466 = Build Path(base path=w1158, name or relative path=w1159) -> (appended path=w1142:path)
          n467 = call <resource>:"Scripting_OpenViRef.vi"("error in"=w1143, "ViPath/ViName/Viref"=w1142, "AppRef"=w1135) -> ("error out"=w1144:errorcluster, "vi reference"=w1140:refnum<vi>)  [unwired: 6 in, 1 out]
          n468 = call <resource>:"GDSLvIcon_AnalyseViIcon.vi"("ViRef/LvCLassRef/LvLibRef/ViPath/2D_Image"=w1140, "error in (no error)"=w1144) -> ("FrameColor"=w1157:u32, "FrameThickness(1)"=w1155:u32, "HeaderIcon"=w1150:u8[][], "HeaderBkColor"=w1145:u32, "BodyBkColor"=w1156:u32, "error out"=w1141:errorcluster)  [unwired: 5 in, 7 out]
          n469 = Array Size(array=w1150) -> (size(s)=w1149:i32[])
          n470 = Close Reference(reference=w1140, error in (no error)=w1141) -> ()  [unwired: 1 out]
          n471 = Index Array(array=w1149) -> (element=w1147:i32)  [unwired: 1 in]
          n472 = Subtract(x=u32 32 ("Width(30)"), y=w1147) -> (x-y=w1146:u32)
          n473 = Multiply(x=w1155, y=u32 2) -> (x*y=w1153:u32)
          n474 = Subtract(x=u32 32 ("Width(30)"), y=w1153) -> (x-y=w1151:u32)
          n475 = call <resource>:"GDSLvIcon_GenerateObjectIcon.vi"("HeaderColor"=w1145, "BackgroundColor"=w1156, "Height"=w1146, "error in (no error)"=w1141, "Type"=enum16{"LvClass", "Library", "X-Control"}."LvClass", "Width(30)"=w1151) -> ("BodyIconOut"=w1162:u8[][], "error out"=w1163:errorcluster)  [unwired: 12 in]
          n476 = call <resource>:"GDSLvIcon_CreateIconPicture.vi"("FrameColor"=w1157, "FrameThickness(1)"=w1155, "HeaderIconIn"=w1150, "BodyIconIn"=w1162, "error in (no error)"=w1163) -> ("WholeIconOut"=w1167:u8[][], "error out"=w1164:errorcluster)  [unwired: 9 in, 4 out]
          n477 = Reshape Array(w1167, 1024 ("dimension size")) -> (w1165:u8[])
          n478 = Bundle By Name(cluster=T12 {"image type"=0, "image depth"=8, "image"=[], "mask"=[], "colors"=[], "Rectangle"={"left"=0, "top"=0, "right"=32, "bottom"=32}} ("image data"), "image"=w1165) -> (w1138:T12)
          n479 = invoke class="LVClassLibrary" method="Set Icon"(reference=w1136, error in=w1164, "color"=w1138) -> (reference out=w1131:refnum<vi>, error out=w1132:errorcluster)  [unwired: 2 in, 3 out]
          n480 = property class="LVClassLibrary"(reference=w1131, error in=w1132) -> (reference out=w1130:refnum<vi>, error out=w1137:errorcluster, "Member Data"=w1139:refnum<vi>)
          n481 = invoke class="VI" method="VI Icon.Set from Image Data"(reference=w1139, error in=w1137, "ImageData"=w1138) -> (reference out=w1133:refnum<vi>, error out=w1134:errorcluster)  [unwired: 3 in, 4 out]
          n482 = Close Reference(reference=w1133, error in (no error)=w1134) -> (error out=w1129:errorcluster)
          n483 = invoke class="LVClassLibrary" method="Save"(reference=w1130, error in=w1129) -> (error out=w1128:errorcluster)  [unwired: 2 in, 3 out]
          n484 = stacked-sequence {
            tunnel: w1128 -> [_]
            frame #0 {
              n485 = Wait (ms)(milliseconds to wait=u32 2) -> ()  [unwired: 1 out]
            }
          }
        }
        n486 = property on="Progress" class="LstBox (strict)"() -> ("Item Names"=w1123:string[], "Number of Rows"=w1117:u32)  [unwired: 2 in, 2 out]
        n487 = Build Array (concatenate)(w1123, string[] ["Updating Icons"] ("element")) -> (w1118:string[])
        n488 = Array Size(array=w1118) -> (size(s)=w1122:i32)
        n489 = Subtract(x=w1122, y=w1117) -> (x-y=w1121:u32)
        n490 = To Long Integer(number=w1121) -> (32bit integer=w1119:i32)
        n491 = Max & Min(x=w1119, y=0) -> (max(x,y)=w1116:i32)  [unwired: 1 out]
        n492 = property on="Progress" class="LstBox (strict)"("Item Names"=w1118, "Top Row"=w1116) -> ()  [unwired: 2 in, 2 out]
        n493 = Unbundle By Name(w1111) -> ("Classes"=w1110:T2[], "VIsToRelink"=w1109:refnum<vi>[])
        n494 = call <resource>:"ConvertGoop2ToGoop3_RecompileAll.vi"("error IO 2"=w1114, "VIsToRelink"=w1109, "Classes"=w1110) -> ("error IO"=w1113:errorcluster)  [unwired: 6 in]
      }
      frame "UpdateLvClassAttributes" {
        n495 = Unbundle By Name(w1174) -> ("Classes"=w1178:T2[])
        n496 = for {
          tunnel: w1178 -> [w1195] mode=indexing
          shift-right: [w1193] -> w1176
          shift-left: w1177 -> [w1193]
          n497 = Unbundle By Name(w1195) -> ("ClassName"=w1180:string, "ClassRef"=w1194:refnum<vi>)
          n498 = call <resource>:"Scripting_PlaceGoopRefInClassAttribute.vi"("error in"=w1193, "ClassRefnum"=w1194) -> ("error out"=w1192:errorcluster, "ClusterTypeDefPath"=w1190:path, "ObjectRef.ctl"=w1191:path)  [unwired: 2 in, 1 out]
          n499 = case shown="No Error" w1192 {
            tunnel: w1180 -> [_ w1201]
            tunnel: w1191 -> [_ w1199]
            tunnel: w1190 -> [_ w1197]
            frame No Error {
              n500 = stacked-sequence {
                frame #0 {
                  n501 = Wait (ms)(milliseconds to wait=u32 2) -> ()  [unwired: 1 out]
                }
              }
            }
            frame Error {
              w1205 = path "c:/G2To3.txt" ("file (use dialog)")
              n502 = Path To String(path=w1197) -> (string=w1198:string)
              n503 = Path To String(path=w1199) -> (string=w1200:string)
              n504 = Read from Text File(file (use dialog)=w1205) -> (text=w1202:string)  [unwired: 3 in, 3 out]
              n505 = Format Into String(format string="       Error %s(%s)%s\n", initial string=w1202, w1201, w1198, w1200) -> (resulting string=w1204:string)  [unwired: 1 in, 1 out]
              n506 = stacked-sequence {
                tunnel: w1204 -> [w1208]
                tunnel: w1205 -> [w1206]
                frame #0 {
                  n507 = Delete(path (use dialog)=w1206) -> (deleted path=w1207:path)  [unwired: 4 in, 2 out]
                  n508 = Write to Text File(file (use dialog)=w1207, text=w1208) -> ()  [unwired: 2 in, 3 out]
                }
              }
              n509 = call <vilib>:"Beep.vi"() -> ()  [unwired: 12 in]
            }
          }
          n510 = Format Into String(format string="Updating LvClass Attribute: %s", w1180) -> (resulting string=w1179:string)  [unwired: 2 in, 1 out]
          n511 = property on="Progress" class="LstBox (strict)"() -> ("Item Names"=w1189:string[], "Number of Rows"=w1183:u32)  [unwired: 2 in, 2 out]
          n512 = Build Array (concatenate)(w1189, w1179) -> (w1184:string[])
          n513 = Array Size(array=w1184) -> (size(s)=w1188:i32)
          n514 = Subtract(x=w1188, y=w1183) -> (x-y=w1187:u32)
          n515 = To Long Integer(number=w1187) -> (32bit integer=w1185:i32)
          n516 = Max & Min(x=w1185, y=0) -> (max(x,y)=w1182:i32)  [unwired: 1 out]
          n517 = property on="Progress" class="LstBox (strict)"("Item Names"=w1184, "Top Row"=w1182) -> ()  [unwired: 2 in, 2 out]
        }
        n518 = Unbundle By Name(w1174) -> ("Classes"=w1173:T2[], "VIsToRelink"=w1172:refnum<vi>[])
        n519 = call <resource>:"ConvertGoop2ToGoop3_RecompileAll.vi"("error IO 2"=w1176, "VIsToRelink"=w1172, "Classes"=w1173) -> ("error IO"=w1175:errorcluster)  [unwired: 6 in]
      }
      frame "UpdateNewCallers" {
        n520 = Unbundle By Name(w1220) -> ("Classes"=w1222:T2[])
        n521 = for {
          tunnel: w1222 -> [w1239] mode=indexing
          shift-right: [w1237] -> w1221
          shift-left: w1219 -> [w1238]
          n522 = Unbundle By Name(w1239) -> ("ViRefs"=w1236:refnum<vi>[], "ClassFolder"=w1235:path, "ClassName"=w1229:string)
          n523 = Concatenate Strings(w1229, "_New.vi" ("string")) -> (w1233:string)
          n524 = Concatenate Strings(w1229, "_GetAttributesToModify.vi" ("string")) -> (w1227:string)
          n525 = Concatenate Strings(w1229, "_SetModifiedAttributes.vi" ("string")) -> (w1224:string)
          n526 = Build Path(base path=w1235, name or relative path="Utils") -> (appended path=w1225:path)
          n527 = Build Path(base path=w1225, name or relative path=w1233) -> (appended path=w1232:path)
          n528 = Build Path(base path=w1225, name or relative path=w1227) -> (appended path=w1226:path)
          n529 = Build Path(base path=w1225, name or relative path=w1224) -> (appended path=w1223:path)
          n530 = for {
            tunnel: w1236 -> [w1243] mode=indexing
            shift-right: [w1245] -> w1237
            shift-left: w1238 -> [w1244]
            tunnel: w1232 -> [w1242]
            tunnel: w1226 -> [w1241]
            tunnel: w1223 -> [w1240]
            n531 = call <resource>:"Scripting_G1NewToG3New.vi"("VI Refnum"=w1243, "SearchVI"=w1242, "GetToModify"=w1241, "SetToModify"=w1240, "error IO"=w1244) -> ("error out"=w1245:errorcluster)  [unwired: 14 in]
          }
        }
        n532 = property on="Progress" class="LstBox (strict)"() -> ("Item Names"=w1218:string[], "Number of Rows"=w1212:u32)  [unwired: 2 in, 2 out]
        n533 = Build Array (concatenate)(w1218, "Update NEW-VI callers") -> (w1213:string[])
        n534 = Array Size(array=w1213) -> (size(s)=w1217:i32)
        n535 = Subtract(x=w1217, y=w1212) -> (x-y=w1216:u32)
        n536 = To Long Integer(number=w1216) -> (32bit integer=w1214:i32)
        n537 = Max & Min(x=w1214, y=0) -> (max(x,y)=w1211:i32)  [unwired: 1 out]
        n538 = property on="Progress" class="LstBox (strict)"("Item Names"=w1213, "Top Row"=w1211) -> ()  [unwired: 2 in, 2 out]
      }
      frame "UpdateDeleteCallers" {
        n539 = Unbundle By Name(w1257) -> ("Classes"=w1259:T2[])
        n540 = for {
          tunnel: w1259 -> [w1273] mode=indexing
          shift-right: [w1271] -> w1258
          shift-left: w1256 -> [w1272]
          n541 = Unbundle By Name(w1273) -> ("ViRefs"=w1270:refnum<vi>[], "ClassFolder"=w1269:path, "ClassName"=w1264:string)
          n542 = Concatenate Strings(w1264, "_Delete.vi" ("string")) -> (w1267:string)
          n543 = Concatenate Strings(w1264, "_GetAttributes.vi" ("string")) -> (w1262:string)
          n544 = Build Path(base path=w1269, name or relative path="Utils") -> (appended path=w1260:path)
          n545 = Build Path(base path=w1260, name or relative path=w1267) -> (appended path=w1266:path)
          n546 = Build Path(base path=w1260, name or relative path=w1262) -> (appended path=w1261:path)
          n547 = for {
            tunnel: w1270 -> [w1276] mode=indexing
            shift-right: [w1278] -> w1271
            shift-left: w1272 -> [w1277]
            tunnel: w1266 -> [w1275]
            tunnel: w1261 -> [w1274]
            n548 = call <resource>:"Scripting_G1DeleteToG3Delete.vi"("VI Refnum"=w1276, "SearchVI"=w1275, "Get"=w1274, "error IO"=w1277) -> ("error out"=w1278:errorcluster)  [unwired: 15 in]
          }
        }
        n549 = property on="Progress" class="LstBox (strict)"() -> ("Item Names"=w1255:string[], "Number of Rows"=w1249:u32)  [unwired: 2 in, 2 out]
        n550 = Build Array (concatenate)(w1255, "Update Delete-VI callers") -> (w1250:string[])
        n551 = Array Size(array=w1250) -> (size(s)=w1254:i32)
        n552 = Subtract(x=w1254, y=w1249) -> (x-y=w1253:u32)
        n553 = To Long Integer(number=w1253) -> (32bit integer=w1251:i32)
        n554 = Max & Min(x=w1251, y=0) -> (max(x,y)=w1248:i32)  [unwired: 1 out]
        n555 = property on="Progress" class="LstBox (strict)"("Item Names"=w1250, "Top Row"=w1248) -> ()  [unwired: 2 in, 2 out]
      }
      frame "UpdateConnectorPane" {
        n556 = Unbundle By Name(w1279) -> ("Classes"=w1292:T2[])
        n557 = for {
          tunnel: w1292 -> [w1297] mode=indexing
          shift-right: [w1295] -> w1281
          shift-left: w1282 -> [w1296]
          n558 = Unbundle By Name(w1297) -> ("ViRefs"=w1294:refnum<vi>[], "ViPathes"=w1293:path[])  [unwired: 1 out]
          n559 = for {
            tunnel: w1294 -> [w1313] mode=indexing
            shift-right: [w1299] -> w1295
            shift-left: w1296 -> [w1300]
            tunnel: w1293 -> [w1312] mode=indexing
            w1307 = u32 4834  # 6+6+6
            n560 = property class="VI"(reference=w1313, error in=w1300) -> (reference out=w1298:refnum<vi>, error out=w1314:errorcluster, "ConPane"=w1315:refnum<vi>)
            n561 = Strip Path(path=w1312) -> (name=w1311:string)  [unwired: 1 out]
            n562 = property class="ConPane"(reference=w1315, error in=w1314) -> (reference out=w1301:refnum<vi>, error out=w1306:errorcluster, "Pattern"=w1308:u32)
            n563 = Match Pattern(string=w1311, regular expression="GOOPKernel.vi") -> (offset past match=w1309:i32)  [unwired: 1 in, 3 out]
            n564 = Less Than 0?(x=w1309) -> (x < 0?=w1303:bool)
            n565 = Not Equal?(x=w1308, y=w1307) -> (x != y?=w1304:bool)
            n566 = Unbundle(w1306) -> ("status"=w1305:bool)  [unwired: 2 out]
            n567 = Compound Arithmetic op=AND(invert w1305, w1304, w1303) -> (w1302:bool)
            n568 = case shown="True" w1302 {
              tunnel: w1301 -> [w1317 w1327]
              tunnel: w1300 -> [w1316 w1319]
              tunnel: [w1316 w1321] -> w1299
              tunnel: w1298 -> [_ w1318]
              frame False {
                n569 = Close Reference(reference=w1317) -> ()  [unwired: 1 in, 1 out]
              }
              frame True {
                w1333 = u32 4826  # 4+1+1+4
                w1330 = u32 4834  # 6+6+6
                n570 = property class="ConPane"(reference=w1327, error in=w1319, "Pattern"=w1333) -> (reference out=w1332:refnum<vi>, error out=w1331:errorcluster)
                n571 = property class="ConPane"(reference=w1332, error in=w1331, "Pattern"=w1330) -> (reference out=w1328:refnum<vi>, error out=w1329:errorcluster)
                n572 = Close Reference(reference=w1328, error in (no error)=w1329) -> (error out=w1320:errorcluster)
                n573 = property class="VI"(reference=w1318, error in=w1320) -> (error out=w1323:errorcluster, "Callers"=w1322:string[], "OwningApp"=w1326:refnum<vi>, "Path"=w1324:path)  [unwired: 1 out]
                n574 = for {
                  tunnel: w1322 -> [w1344] mode=indexing
                  tunnel: w1324 -> [w1341]
                  tunnel: w1326 -> [w1337]
                  shift-right: [w1334] -> w1325
                  shift-left: w1323 -> [w1343]
                  n575 = Build Array(w1341) -> (w1340:path[])
                  n576 = call <resource>:"Scripting_OpenViRef.vi"("error in"=w1343, "ViPath/ViName/Viref"=w1344, "AppRef"=w1337) -> ("error out"=w1342:errorcluster, "vi reference"=w1335:refnum<vi>)  [unwired: 6 in, 1 out]
                  n577 = call <resource>:"Scripting_FindVisOnDiagram.vi"("ViRef"=w1335, "VIsToSerachFor/ViName"=w1340, "error in (no error)"=w1342) -> ("VisFound"=w1338:refnum<vi>[], "error out"=w1339:errorcluster)  [unwired: 15 in]
                  n578 = for {
                    tunnel: w1338 -> [w1351] mode=indexing
                    shift-right: [w1347] -> w1336
                    shift-left: w1339 -> [w1350]
                    n579 = To More Specific Class(target class=refnum<vi> refnum ("WhileLoop"), reference=w1351, error in=w1350) -> (specific class reference=w1349:refnum<vi>, error out=w1348:errorcluster)
                    n580 = invoke class="SubVI" method="Relink To VI"(reference=w1349, error in=w1348) -> (error out=w1347:errorcluster, "Relink To VI"=w1346:refnum<vi>)  [unwired: 1 in, 1 out]
                    n581 = Close Reference(reference=w1346, error in (no error)=w1347) -> ()  [unwired: 1 out]
                  }
                  n582 = Close Reference(reference=w1335, error in (no error)=w1336) -> (error out=w1334:errorcluster)
                  n583 = for {
                    tunnel: w1338 -> [w1345] mode=indexing
                    tunnel: w1334 -> [_]
                    n584 = Close Reference(reference=w1345) -> ()  [unwired: 1 in, 1 out]
                  }
                }
                n585 = Close Reference(reference=w1326, error in (no error)=w1325) -> (error out=w1321:errorcluster)
              }
            }
          }
        }
        n586 = property on="Progress" class="LstBox (strict)"() -> ("Item Names"=w1291:string[], "Number of Rows"=w1285:u32)  [unwired: 2 in, 2 out]
        n587 = Build Array (concatenate)(w1291, "Update ConnectorPane") -> (w1286:string[])
        n588 = Array Size(array=w1286) -> (size(s)=w1290:i32)
        n589 = Subtract(x=w1290, y=w1285) -> (x-y=w1289:u32)
        n590 = To Long Integer(number=w1289) -> (32bit integer=w1287:i32)
        n591 = Max & Min(x=w1287, y=0) -> (max(x,y)=w1284:i32)  [unwired: 1 out]
        n592 = property on="Progress" class="LstBox (strict)"("Item Names"=w1286, "Top Row"=w1284) -> ()  [unwired: 2 in, 2 out]
      }
      frame "UpdateClassInfo" {
        n593 = Unbundle By Name(w1364) -> ("Classes"=w1367:T2[], "TemplateVersions"=w1353:string[])
        n594 = for {
          tunnel: w1367 -> [w1372] mode=indexing
          shift-right: [w1369] -> w1365
          shift-left: w1366 -> [w1377]
          tunnel: w1353 -> [w1368] mode=indexing
          n595 = Unbundle By Name(w1372) -> ("InheritsFrom"=w1376:path)
          n596 = Unbundle By Name(w1372) -> ("ClassRef"=w1370:refnum<vi>)
          n597 = property class="LVClassLibrary"(reference=w1370, error in=w1377) -> (reference out=w1384:refnum<vi>, error out=w1385:errorcluster, "Description"=w1383:string)
          n598 = Empty String/Path?(string/path=w1376) -> (empty?=w1375:bool)
          n599 = Select(t=EndevoTemplateNames."BaseTemplate" ("TemplateNames"), s=w1375, f=EndevoTemplateNames."SubTemplate" ("TemplateNames")) -> (s? t:f=w1371:T9)
          n600 = Format Into String(w1371) -> (resulting string=w1382:string)  [unwired: 3 in, 1 out]
          n601 = Format Into String(EndevoProviderName."EndevoGOOP300" ("ProviderName")) -> (resulting string=w1381:string)  [unwired: 3 in, 1 out]
          n602 = Bundle By Name(cluster=T3 {"ClassProviderName"="", "ClassTemplateUsed"="", "ClassTemplateVersion"="", "ClassDescription"="", "PlugIns"=[], "ConnectorPanePattern"=""} ("ClassSettings"), "ClassProviderName"=w1381, "ClassTemplateUsed"=w1382, "ClassTemplateVersion"=w1368, "ClassDescription"=w1383) -> (w1379:T3)
          n603 = call <resource>:"GDSLvClass_StoreClassType.vi"("Class Refnum In"=w1384, "ClassSettings"=w1379, "error in (no error)"=w1385) -> ("error out"=w1369:errorcluster)  [unwired: 15 in, 1 out]
          n604 = stacked-sequence {
            tunnel: w1369 -> [_]
            frame #0 {
              n605 = Wait (ms)(milliseconds to wait=u32 5) -> ()  [unwired: 1 out]
            }
          }
        }
        n606 = property on="Progress" class="LstBox (strict)"() -> ("Item Names"=w1362:string[], "Number of Rows"=w1356:u32)  [unwired: 2 in, 2 out]
        n607 = Build Array (concatenate)(w1362, "Update class info") -> (w1357:string[])
        n608 = Array Size(array=w1357) -> (size(s)=w1361:i32)
        n609 = Subtract(x=w1361, y=w1356) -> (x-y=w1360:u32)
        n610 = To Long Integer(number=w1360) -> (32bit integer=w1358:i32)
        n611 = Max & Min(x=w1358, y=0) -> (max(x,y)=w1355:i32)  [unwired: 1 out]
        n612 = property on="Progress" class="LstBox (strict)"("Item Names"=w1357, "Top Row"=w1355) -> ()  [unwired: 2 in, 2 out]
      }
    }
    n613 = call <vilib>:"Clear Errors.vi"("error in (no error)"=w19) -> ("error out"=w18:errorcluster)  [unwired: 5 in, 1 out]
    n614 = Equal?(x=w29, y="Exit") -> (x = y?=w32:bool)
    n615 = Select(t="Error", s=w18, f=w29) -> (s? t:f=w33:string)
    "State" <- w23
  }
  n616 = Unbundle By Name(w13) -> ("error"=w10:errorcluster)
  n617 = call <resource>:"GDSError_ReportError.vi"("error in (no error)"=w10) -> ("error out"=w4:errorcluster)  [unwired: 18 in]
  "error out" <- w4
  n618 = property class="VI"(reference=w2, error in=w4, "Front Panel.Open"=FALSE ("Front Panel Window:Open")) -> (reference out=w1:refnum<vi>, error out=w3:errorcluster)
  n619 = Close Reference(reference=w1, error in (no error)=w3) -> ()  [unwired: 1 out]
